vi "Batch_main_with_graph.vi"(1 "Stop":bool, 2 "ExpFilePath":path=path "D:/BaptisteData/BM13/CD1/data1/stabRF_exp_38.h5") -> ()   [LabVIEW 2013]
uses:
  <vilib>/addons/h5labview2/base/hid_t.ctl
  fpga-bitfile-ref.ctl
  host-subvis/Fast_sequence/sequence slot/slot-use.ctl
  host-subvis/Fast_sequence/sequence slot/triggers.ctl
  host-subvis/Fast_sequence/sequence slot/DAC.ctl
  host-subvis/Fast_sequence/sequence slot/DAC_fastseq-offset.ctl
  host-subvis/Fast_sequence/sequence slot/timing.ctl
  host-subvis/Fast_sequence/sequence slot/jump.ctl
  <vilib>/addons/h5labview2/file/H5Fmode.ctl
  <vilib>/addons/h5labview2/base/lib_path.vi
  <vilib>/addons/h5labview2/base/H5Equery.vi
  <vilib>/FPGAPlugInAG/sbRIO-9612/niLvFpga_Close_sbRIO-9612.vi
  <vilib>/addons/h5labview2/dataset/H5Dread.llb/H5Dread.xnode
  <vilib>/addons/h5labview2/attrib/H5Aread.llb/H5Aread.xnode
  <vilib>/rvi/interface/nirviCloseFPGA/nirviCloseFPGA.xnode
  FPGA Bitfiles/fpgabatch18_sbRIO9612RIO0_FPGAMAINMerlin_-1tLGtxjYvQ.lvbitx
  <vilib>/addons/h5labview2/attrib/H5Awrite.llb/H5Awrite.xnode
  <vilib>/addons/h5labview2/file/H5F.lvlib
  <vilib>/addons/h5labview2/dataset/H5D.lvlib
  <vilib>/addons/h5labview2/space/H5S.lvlib
panel:
  out "Remaning time (min)":dbl
  in  "temp file interval (ms)":i32=600
  in  "get variable interval (ms)":i32=300
  out "Graph":T1(graph)
  in  "Plot parameters":T2
  out "Temp data":sgl[][](array[numeric])
  out "Initial positions":T3(array[cluster])=[{"Name"="AWG", "kind"=7, "Value"=0.0}, {"Name"="Freq", "kind"=6, "Value"=2759965000.0}, {"Name"="Power", "kind"=6, "Value"=-40.0}, {"Name"="sus", "kind"=4, "Value"=0.29998779296875}, {"Name"="rus", "kind"=4, "Value"=0.29998779296875}, {"Name"="rls", "kind"=4, "Value"=0.29998779296875}, {"Name"="sls", "kind"=4, "Value"=0.059967041015625}, {"Name"="suq", "kind"=4, "Value"=-1.75994873046875}, {"Name"="suu", "kind"=4, "Value"=-0.749969482421875}, {"Name"="sur", "kind"=4, "Value"=-1.199951171875}, {"Name"="suc", "kind"=4, "Value"=-0.449981689453125}, {"Name"="sul", "kind"=4, "Value"=-0.89996337890625}, {"Name"="ruq", "kind"=4, "Value"=-1.699981689453125}, {"Name"="ruu", "kind"=4, "Value"=-0.749969482421875}, {"Name"="rur", "kind"=4, "Value"=-1.25}, {"Name"="ruc", "kind"=4, "Value"=-0.399932861328125}, {"Name"="rul", "kind"=4, "Value"=-0.89996337890625}, {"Name"="rlq", "kind"=4, "Value"=-1.7999267578125}, {"Name"="rlu", "kind"=4, "Value"=-0.89996337890625}, {"Name"="rlr", "kind"=4, "Value"=-1.199951171875}, {"Name"="rlc", "kind"=4, "Value"=-0.5999755859375}, {"Name"="rll", "kind"=4, "Value"=-0.749969482421875}, {"Name"="slq", "kind"=4, "Value"=-1.62506103515625}, {"Name"="slu", "kind"=4, "Value"=-0.89996337890625}, {"Name"="slr", "kind"=4, "Value"=-1.150054931640625}, {"Name"="slc", "kind"=4, "Value"=-0.449981689453125}, {"Name"="sll", "kind"=4, "Value"=-0.749969482421875}, {"Name"="tu", "kind"=4, "Value"=-0.89996337890625}, {"Name"="t", "kind"=4, "Value"=-0.89996337890625}, {"Name"="tl", "kind"=4, "Value"=-0.89996337890625}, {"Name"="4:7", "kind"=4, "Value"=-1.00006103515625}]
  in  "Buf size":i32=300
  out "Var index":u64[](array[numeric])=[0, 49, 0]
  out "start read vals":bool=TRUE
  out "Indexes File":u64[](array[numeric])=[8, 21, 0]
  out "Finish":bool=TRUE
  out "error out":errorcluster
  in  "File update interval (sec)":i32=3000000
  out "DAC_lock-in_info":T4={"Kind"=5, "Strings"=["DAC_Lock-in", "10.0.0.2", "V"], "uint64s"=[0, 1, 0, 0], "Doubles"=[1.0, 0.0, -1.0, -1.0, 50.0, 0.10000000149011612], "DAQmx take out list"=[]}
  out "Fast sequence parameters":T11={"Sequence size"=22, "IP address"="10.0.0.2", "Fast-seq-divider"=6661, "Trigger length"=300, "Sample count"=100, "Send all points?"=FALSE, "Upper limit"=1.0, "Lower limit"=-1.0, "Start ramp at"=0, "fast channels"=[{"dummy?"=FALSE, "panel"=0, "channel"=7}, {"dummy?"=FALSE, "panel"=1, "channel"=0}, {"dummy?"=FALSE, "panel"=0, "channel"=5}, {"dummy?"=FALSE, "panel"=1, "channel"=5}, {"dummy?"=FALSE, "panel"=1, "channel"=6}, {"dummy?"=FALSE, "panel"=1, "channel"=2}, {"dummy?"=FALSE, "panel"=2, "channel"=2}, {"dummy?"=FALSE, "panel"=2, "channel"=3}, {"dummy?"=FALSE, "panel"=2, "channel"=0}, {"dummy?"=FALSE, "panel"=2, "channel"=7}, {"dummy?"=FALSE, "panel"=3, "channel"=0}, {"dummy?"=FALSE, "panel"=2, "channel"=5}, {"dummy?"=FALSE, "panel"=3, "channel"=2}, {"dummy?"=FALSE, "panel"=3, "channel"=3}, {"dummy?"=FALSE, "panel"=3, "channel"=4}, {"dummy?"=FALSE, "panel"=4, "channel"=7}], "fastseq"=[{"use"=enum."triggers", "Triggers"={"triggers"={"1"=TRUE, "2"=TRUE, "3"=FALSE, "4"=FALSE}, "stop"=FALSE}, "DAC"={"FastChanNum"=0, "DAC offset"=0.0}, "timing"=0.0, "slot#"=0}, {"use"=enum."timing", "Triggers"={"triggers"={"1"=FALSE, "2"=FALSE, "3"=FALSE, "4"=FALSE}, "stop"=FALSE}, "DAC"={"FastChanNum"=0, "DAC offset"=0.0}, "timing"=1.0, "slot#"=0}, {"use"=enum."triggers", "Triggers"={"triggers"={"1"=TRUE, "2"=FALSE, "3"=FALSE, "4"=FALSE}, "stop"=FALSE}, "DAC"={"FastChanNum"=0, "DAC offset"=0.0}, "timing"=0.0, "slot#"=0}, {"use"=enum."timing", "Triggers"={"triggers"={"1"=FALSE, "2"=FALSE, "3"=FALSE, "4"=FALSE}, "stop"=FALSE}, "DAC"={"FastChanNum"=0, "DAC offset"=0.0}, "timing"=1.0, "slot#"=0}, {"use"=enum."DAC", "Triggers"={"triggers"={"1"=FALSE, "2"=FALSE, "3"=FALSE, "4"=FALSE}, "stop"=FALSE}, "DAC"={"FastChanNum"=1, "DAC offset"=0.0}, "timing"=0.0, "slot#"=0}, {"use"=enum."DAC", "Triggers"={"triggers"={"1"=FALSE, "2"=FALSE, "3"=FALSE, "4"=FALSE}, "stop"=FALSE}, "DAC"={"FastChanNum"=0, "DAC offset"=0.0}, "timing"=0.0, "slot#"=0}, {"use"=enum."DAC", "Triggers"={"triggers"={"1"=FALSE, "2"=FALSE, "3"=FALSE, "4"=FALSE}, "stop"=FALSE}, "DAC"={"FastChanNum"=4, "DAC offset"=0.0}, "timing"=0.0, "slot#"=0}, {"use"=enum."DAC", "Triggers"={"triggers"={"1"=FALSE, "2"=FALSE, "3"=FALSE, "4"=FALSE}, "stop"=FALSE}, "DAC"={"FastChanNum"=3, "DAC offset"=0.0}, "timing"=0.0, "slot#"=0}, {"use"=enum."DAC", "Triggers"={"triggers"={"1"=FALSE, "2"=FALSE, "3"=FALSE, "4"=FALSE}, "stop"=FALSE}, "DAC"={"FastChanNum"=7, "DAC offset"=0.0}, "timing"=0.0, "slot#"=0}, {"use"=enum."DAC", "Triggers"={"triggers"={"1"=FALSE, "2"=FALSE, "3"=FALSE, "4"=FALSE}, "stop"=FALSE}, "DAC"={"FastChanNum"=6, "DAC offset"=0.0}, "timing"=0.0, "slot#"=0}, {"use"=enum."DAC", "Triggers"={"triggers"={"1"=FALSE, "2"=FALSE, "3"=FALSE, "4"=FALSE}, "stop"=FALSE}, "DAC"={"FastChanNum"=10, "DAC offset"=0.0}, "timing"=0.0, "slot#"=0}, {"use"=enum."DAC", "Triggers"={"triggers"={"1"=FALSE, "2"=FALSE, "3"=FALSE, "4"=FALSE}, "stop"=FALSE}, "DAC"={"FastChanNum"=9, "DAC offset"=0.0}, "timing"=0.0, "slot#"=0}, {"use"=enum."timing", "Triggers"={"triggers"={"1"=FALSE, "2"=FALSE, "3"=FALSE, "4"=FALSE}, "stop"=FALSE}, "DAC"={"FastChanNum"=0, "DAC offset"=0.0}, "timing"=10.0, "slot#"=0}, {"use"=enum."DAC", "Triggers"={"triggers"={"1"=FALSE, "2"=FALSE, "3"=FALSE, "4"=FALSE}, "stop"=FALSE}, "DAC"={"FastChanNum"=1, "DAC offset"=0.0}, "timing"=0.0, "slot#"=0}, {"use"=enum."DAC", "Triggers"={"triggers"={"1"=FALSE, "2"=FALSE, "3"=FALSE, "4"=FALSE}, "stop"=FALSE}, "DAC"={"FastChanNum"=0, "DAC offset"=0.0}, "timing"=0.0, "slot#"=0}, {"use"=enum."DAC", "Triggers"={"triggers"={"1"=FALSE, "2"=FALSE, "3"=FALSE, "4"=FALSE}, "stop"=FALSE}, "DAC"={"FastChanNum"=4, "DAC offset"=0.0}, "timing"=0.0, "slot#"=0}, {"use"=enum."DAC", "Triggers"={"triggers"={"1"=FALSE, "2"=FALSE, "3"=FALSE, "4"=FALSE}, "stop"=FALSE}, "DAC"={"FastChanNum"=3, "DAC offset"=0.0}, "timing"=0.0, "slot#"=0}, {"use"=enum."DAC", "Triggers"={"triggers"={"1"=FALSE, "2"=FALSE, "3"=FALSE, "4"=FALSE}, "stop"=FALSE}, "DAC"={"FastChanNum"=7, "DAC offset"=0.0}, "timing"=0.0, "slot#"=0}, {"use"=enum."DAC", "Triggers"={"triggers"={"1"=FALSE, "2"=FALSE, "3"=FALSE, "4"=FALSE}, "stop"=FALSE}, "DAC"={"FastChanNum"=6, "DAC offset"=0.0}, "timing"=0.0, "slot#"=0}, {"use"=enum."DAC", "Triggers"={"triggers"={"1"=FALSE, "2"=FALSE, "3"=FALSE, "4"=FALSE}, "stop"=FALSE}, "DAC"={"FastChanNum"=10, "DAC offset"=0.0}, "timing"=0.0, "slot#"=0}, {"use"=enum."DAC", "Triggers"={"triggers"={"1"=FALSE, "2"=FALSE, "3"=FALSE, "4"=FALSE}, "stop"=FALSE}, "DAC"={"FastChanNum"=9, "DAC offset"=0.0}, "timing"=0.0, "slot#"=0}, {"use"=enum."jump", "Triggers"={"triggers"={"1"=FALSE, "2"=FALSE, "3"=FALSE, "4"=FALSE}, "stop"=FALSE}, "DAC"={"FastChanNum"=0, "DAC offset"=0.0}, "timing"=0.0, "slot#"=21}]} {"fastseq"."DAC"."DAC offset" min=-1 max=0.5; "fastseq"."DAC"."FastChanNum" max=15 step=1; "fastseq"."slot#" max=4095}
  out "Timings":dbl[][](array[numeric])=[[2417234066.0, 52858.0]] format="%^#_4g"
  out "Indexes":i32[](array[numeric])=[8, 21, 0]
  out "sweep_dim":u64[](array[numeric])=[11, 61, 61]
  out "Readout parameters":T12(array[cluster])=[{"Kind"=0, "Strings"=["ADC", "", "V", "sud;rud;rld;sld", "nA;nA;nA;nA", "100.0;100.0;100.0;100.0"], "uint64s"=[5, 4, 250000, 1, 100, 10106, 1000000, 10000, 0, 1], "Doubles"=[1.0], "DAQmx take out list"=["", ""]}]
  out "Exp_params":T15={"filename"="201612181913", "ExpFilePath"=path "C:/Documents and Settings/Bauerle/Mes documents/takada/HBT6/201612181913.h5", "File Ref list"=[16777217, 33554433, 16777216, 33554432], "sweep_dim"=[11, 61, 61], "sweep_list"=["suq", "ruq", "rlq", "slq", "sur", "rur", "rlr", "slr", "suc", "ruc", "rlc", "slc"], "readout_list"=["sud", "rud", "rld", "sld"], "Sweep instrument bools"=[[0, 0], [0, 0], [0, 0], [0, 0], [0, 0], [0, 0], [0, 0], [0, 0], [0, 0], [0, 0], [0, 0], [0, 0], [0, 0], [0, 0], [0, 0], [0, 0], [0, 0], [0, 0], [0, 0], [0, 0], [0, 0], [0, 0], [0, 0], [0, 0], [0, 0], [0, 0], [0, 0], [0, 0], [0, 0], [0, 0], [0, 0], [0, 0], [0, 0], [0, 0], [0, 0], [0, 0], [0, 0], [0, 0], [0, 0], [0, 0], [0, 0]], "Read out instrument bools"=[[1, 0]], "Experimental bool list"=[TRUE, TRUE], "Initial move"=[{"Name"="None", "kind"=100, "Value"=0.0}], "FPGA Ref"=refnum, "Inst_parameters"={"ConfigFilePath"=path "\\\\10.0.0.7\\takada2/DATA/HBT6/data/Configs/conf_20161218_fc_load.h5", "Inst_list"=["ADC", "AWG", "Freq", "Power", "sus", "rus", "rls", "sls", "suq", "suu", "sur", "suc", "sul", "ruq", "ruu", "rur", "ruc", "rul", "rlq", "rlu", "rlr", "rlc", "rll", "slq", "slu", "slr", "slc", "sll", "tu", "t", "tl", "fast_sequence", "4:7", "suc_load", "sur_load", "ruc_load", "rur_load", "rlc_load", "rlr_load", "slc_load", "slr_load", "load_time"], "fast_mode"=[1, 0], "Wait_times"=[1, 1, 1, 1], "Inst_array"=[{"Kind"=0, "Strings"=["ADC", "", "V", "sud;rud;rld;sld", "nA;nA;nA;nA", "100.0;100.0;100.0;100.0"], "uint64s"=[5, 4, 250000, 1, 100, 10106, 1000000, 1, 0, 1], "Doubles"=[1.0], "DAQmx take out list"=[]}, {"Kind"=7, "Strings"=["AWG", "10.0.0.4", "", "C:\\Documents and Settings\\Bauerle\\Mes documents\\Bautze\\FPGA-clean_works_1.13.6_batchtest\\Python\\AWG", "dummy", "SAWnstrig_v4.py"], "uint64s"=[2, 0, 0, 3, 0, 0, 0, 0, 0, 0, 0, 0, 0, 0], "Doubles"=[1200000000.0, 1.0, 0.0, 1.0, 0.0, 1.0, 0.0, 1.0, 0.0, 1.0, 0.0, 1.0, 0.0], "DAQmx take out list"=[]}, {"Kind"=6, "Strings"=["Freq", "0:19", "GHz"], "uint64s"=[1, 0, 0, 0, 2, 0, 0, 0], "Doubles"=[2.0, -30.0, 200.0, 100.0, 0.0, 6.000999927520752, 9.000000318337698e-06, 30.0, -145.0], "DAQmx take out list"=[]}, {"Kind"=6, "Strings"=["Power", "0:19", "GHz"], "uint64s"=[1, 0, 1, 0, 2, 0, 0, 1], "Doubles"=[2.0, -30.0, 200.0, 100.0, 0.0, 6.000999927520752, 9.000000318337698e-06, 30.0, -145.0], "DAQmx take out list"=[]}, {"Kind"=4, "Strings"=["sus", "10.0.0.2", "mV"], "uint64s"=[0, 1], "Doubles"=[1.0, -1.0, 1.0, -1.0, 1.0], "DAQmx take out list"=[]}, {"Kind"=4, "Strings"=["rus", "10.0.0.2", "mV"], "uint64s"=[0, 2], "Doubles"=[1.0, -1.0, 1.0, -1.0, 1.0], "DAQmx take out list"=[]}, {"Kind"=4, "Strings"=["rls", "10.0.0.2", "mV"], "uint64s"=[0, 3], "Doubles"=[1.0, -1.0, 1.0, -1.0, 1.0], "DAQmx take out list"=[]}, {"Kind"=4, "Strings"=["sls", "10.0.0.2", "mV"], "uint64s"=[0, 4], "Doubles"=[1.0, -1.0, 1.0, -1.0, 1.0], "DAQmx take out list"=[]}, {"Kind"=4, "Strings"=["suq", "10.0.0.2", "V"], "uint64s"=[0, 5], "Doubles"=[0.30000001192092896, -2.0, 1.0, -1.0, 1.0], "DAQmx take out list"=[]}, {"Kind"=4, "Strings"=["suu", "10.0.0.2", "V"], "uint64s"=[0, 6], "Doubles"=[0.30000001192092896, -2.0, 1.0, -1.0, 1.0], "DAQmx take out list"=[]}, {"Kind"=4, "Strings"=["sur", "10.0.0.2", "V"], "uint64s"=[0, 7], "Doubles"=[0.30000001192092896, -2.0, 1.0, -1.0, 1.0], "DAQmx take out list"=[]}, {"Kind"=4, "Strings"=["suc", "10.0.0.2", "V"], "uint64s"=[1, 0], "Doubles"=[0.30000001192092896, -2.0, 1.0, -1.0, 1.0], "DAQmx take out list"=[]}, {"Kind"=4, "Strings"=["sul", "10.0.0.2", "V"], "uint64s"=[1, 1], "Doubles"=[0.30000001192092896, -2.0, 1.0, -1.0, 1.0], "DAQmx take out list"=[]}, {"Kind"=4, "Strings"=["ruq", "10.0.0.2", "V"], "uint64s"=[1, 2], "Doubles"=[0.30000001192092896, -2.0, 1.0, -1.0, 1.0], "DAQmx take out list"=[]}, {"Kind"=4, "Strings"=["ruu", "10.0.0.2", "V"], "uint64s"=[1, 3], "Doubles"=[0.30000001192092896, -2.0, 1.0, -1.0, 1.0], "DAQmx take out list"=[]}, {"Kind"=4, "Strings"=["rur", "10.0.0.2", "V"], "uint64s"=[1, 5], "Doubles"=[0.30000001192092896, -2.0, 1.0, -1.0, 1.0], "DAQmx take out list"=[]}, {"Kind"=4, "Strings"=["ruc", "10.0.0.2", "V"], "uint64s"=[1, 6], "Doubles"=[0.30000001192092896, -2.0, 1.0, -1.0, 1.0], "DAQmx take out list"=[]}, {"Kind"=4, "Strings"=["rul", "10.0.0.2", "V"], "uint64s"=[1, 7], "Doubles"=[0.30000001192092896, -2.0, 1.0, -1.0, 1.0], "DAQmx take out list"=[]}, {"Kind"=4, "Strings"=["rlq", "10.0.0.2", "V"], "uint64s"=[2, 0], "Doubles"=[0.30000001192092896, -2.0, 1.0, -1.0, 1.0], "DAQmx take out list"=[]}, {"Kind"=4, "Strings"=["rlu", "10.0.0.2", "V"], "uint64s"=[2, 1], "Doubles"=[0.30000001192092896, -2.0, 1.0, -1.0, 1.0], "DAQmx take out list"=[]}, {"Kind"=4, "Strings"=["rlr", "10.0.0.2", "V"], "uint64s"=[2, 2], "Doubles"=[0.30000001192092896, -2.0, 1.0, -1.0, 1.0], "DAQmx take out list"=[]}, {"Kind"=4, "Strings"=["rlc", "10.0.0.2", "V"], "uint64s"=[2, 3], "Doubles"=[0.30000001192092896, -2.0, 1.0, -1.0, 1.0], "DAQmx take out list"=[]}, {"Kind"=4, "Strings"=["rll", "10.0.0.2", "V"], "uint64s"=[2, 4], "Doubles"=[0.30000001192092896, -2.0, 1.0, -1.0, 1.0], "DAQmx take out list"=[]}, {"Kind"=4, "Strings"=["slq", "10.0.0.2", "V"], "uint64s"=[2, 5], "Doubles"=[0.30000001192092896, -2.0, 1.0, -1.0, 1.0], "DAQmx take out list"=[]}, {"Kind"=4, "Strings"=["slu", "10.0.0.2", "V"], "uint64s"=[2, 6], "Doubles"=[0.30000001192092896, -2.0, 1.0, -1.0, 1.0], "DAQmx take out list"=[]}, {"Kind"=4, "Strings"=["slr", "10.0.0.2", "V"], "uint64s"=[2, 7], "Doubles"=[0.30000001192092896, -2.0, 1.0, -1.0, 1.0], "DAQmx take out list"=[]}, {"Kind"=4, "Strings"=["slc", "10.0.0.2", "V"], "uint64s"=[3, 0], "Doubles"=[0.30000001192092896, -2.0, 1.0, -1.0, 1.0], "DAQmx take out list"=[]}, {"Kind"=4, "Strings"=["sll", "10.0.0.2", "V"], "uint64s"=[3, 1], "Doubles"=[0.30000001192092896, -2.0, 1.0, -1.0, 1.0], "DAQmx take out list"=[]}, {"Kind"=4, "Strings"=["tu", "10.0.0.2", "V"], "uint64s"=[3, 2], "Doubles"=[0.30000001192092896, -2.0, 1.0, -1.0, 1.0], "DAQmx take out list"=[]}, {"Kind"=4, "Strings"=["t", "10.0.0.2", "V"], "uint64s"=[3, 3], "Doubles"=[0.30000001192092896, -2.0, 1.0, -1.0, 1.0], "DAQmx take out list"=[]}, {"Kind"=4, "Strings"=["tl", "10.0.0.2", "V"], "uint64s"=[3, 4], "Doubles"=[0.30000001192092896, -2.0, 1.0, -1.0, 1.0], "DAQmx take out list"=[]}, {"Kind"=9, "Strings"=["fast_sequence", "10.0.0.2", "V"], "uint64s"=[6661, 300, 100, 0, 7, 8, 5, 13, 14, 10, 18, 19, 16, 23, 24, 21, 26, 27, 28, 39, 0], "Doubles"=[1.0, -1.0, -1.0, -1.0], "DAQmx take out list"=[]}, {"Kind"=4, "Strings"=["4:7", "10.0.0.2", "V"], "uint64s"=[4, 7], "Doubles"=[0.30000001192092896, -2.0, 1.0, -1.0, 1.0], "DAQmx take out list"=[]}, {"Kind"=10, "Strings"=["suc_load", "10.0.0.2", "V"], "uint64s"=[4, 0], "Doubles"=[0.5, -0.5], "DAQmx take out list"=[]}, {"Kind"=10, "Strings"=["sur_load", "10.0.0.2", "V"], "uint64s"=[5, 0], "Doubles"=[0.5, -0.5], "DAQmx take out list"=[]}, {"Kind"=10, "Strings"=["ruc_load", "10.0.0.2", "V"], "uint64s"=[6, 0], "Doubles"=[0.5, -0.5], "DAQmx take out list"=[]}, {"Kind"=10, "Strings"=["rur_load", "10.0.0.2", "V"], "uint64s"=[7, 0], "Doubles"=[0.5, -0.5], "DAQmx take out list"=[]}, {"Kind"=10, "Strings"=["rlc_load", "10.0.0.2", "V"], "uint64s"=[8, 0], "Doubles"=[0.5, -0.5], "DAQmx take out list"=[]}, {"Kind"=10, "Strings"=["rlr_load", "10.0.0.2", "V"], "uint64s"=[9, 0], "Doubles"=[0.5, -0.5], "DAQmx take out list"=[]}, {"Kind"=10, "Strings"=["slc_load", "10.0.0.2", "V"], "uint64s"=[10, 0], "Doubles"=[0.5, -0.5], "DAQmx take out list"=[]}, {"Kind"=10, "Strings"=["slr_load", "10.0.0.2", "V"], "uint64s"=[11, 0], "Doubles"=[0.5, -0.5], "DAQmx take out list"=[]}, {"Kind"=10, "Strings"=["load_time", "10.0.0.2", "ms"], "uint64s"=[12, 0], "Doubles"=[1000.0, -0.009999999776482582], "DAQmx take out list"=[]}]}} {"File Ref list" format="%.0x"}
  out "Sweep inst info":T12(array[cluster])=[{"Kind"=4, "Strings"=["suq", "10.0.0.2", "V"], "uint64s"=[0, 5], "Doubles"=[0.30000001192092896, -2.0, 1.0, -1.0, 1.0], "DAQmx take out list"=[]}, {"Kind"=4, "Strings"=["ruq", "10.0.0.2", "V"], "uint64s"=[1, 2], "Doubles"=[0.30000001192092896, -2.0, 1.0, -1.0, 1.0], "DAQmx take out list"=[]}, {"Kind"=4, "Strings"=["rlq", "10.0.0.2", "V"], "uint64s"=[2, 0], "Doubles"=[0.30000001192092896, -2.0, 1.0, -1.0, 1.0], "DAQmx take out list"=[]}, {"Kind"=4, "Strings"=["slq", "10.0.0.2", "V"], "uint64s"=[2, 5], "Doubles"=[0.30000001192092896, -2.0, 1.0, -1.0, 1.0], "DAQmx take out list"=[]}, {"Kind"=4, "Strings"=["sur", "10.0.0.2", "V"], "uint64s"=[0, 7], "Doubles"=[0.30000001192092896, -2.0, 1.0, -1.0, 1.0], "DAQmx take out list"=[]}, {"Kind"=4, "Strings"=["rur", "10.0.0.2", "V"], "uint64s"=[1, 5], "Doubles"=[0.30000001192092896, -2.0, 1.0, -1.0, 1.0], "DAQmx take out list"=[]}, {"Kind"=4, "Strings"=["rlr", "10.0.0.2", "V"], "uint64s"=[2, 2], "Doubles"=[0.30000001192092896, -2.0, 1.0, -1.0, 1.0], "DAQmx take out list"=[]}, {"Kind"=4, "Strings"=["slr", "10.0.0.2", "V"], "uint64s"=[2, 7], "Doubles"=[0.30000001192092896, -2.0, 1.0, -1.0, 1.0], "DAQmx take out list"=[]}, {"Kind"=4, "Strings"=["suc", "10.0.0.2", "V"], "uint64s"=[1, 0], "Doubles"=[0.30000001192092896, -2.0, 1.0, -1.0, 1.0], "DAQmx take out list"=[]}, {"Kind"=4, "Strings"=["ruc", "10.0.0.2", "V"], "uint64s"=[1, 6], "Doubles"=[0.30000001192092896, -2.0, 1.0, -1.0, 1.0], "DAQmx take out list"=[]}, {"Kind"=4, "Strings"=["rlc", "10.0.0.2", "V"], "uint64s"=[2, 3], "Doubles"=[0.30000001192092896, -2.0, 1.0, -1.0, 1.0], "DAQmx take out list"=[]}, {"Kind"=4, "Strings"=["slc", "10.0.0.2", "V"], "uint64s"=[3, 0], "Doubles"=[0.30000001192092896, -2.0, 1.0, -1.0, 1.0], "DAQmx take out list"=[]}]
  # "total"
  # "nb of calls"
  # "average"
  # "total time"
  # "read config"
  # "plot loop"
  # "save data"
  # "config instr"
  # "FPGA init"
  # "voltmeter init"
  # "initial move"
  # "read init values"
  # "meas loop"
  # "move + wait"
  # "FPGA config"
  # "FPGA start"
  # "FPGA stop"
  # "read data"
  # "clear buffer"
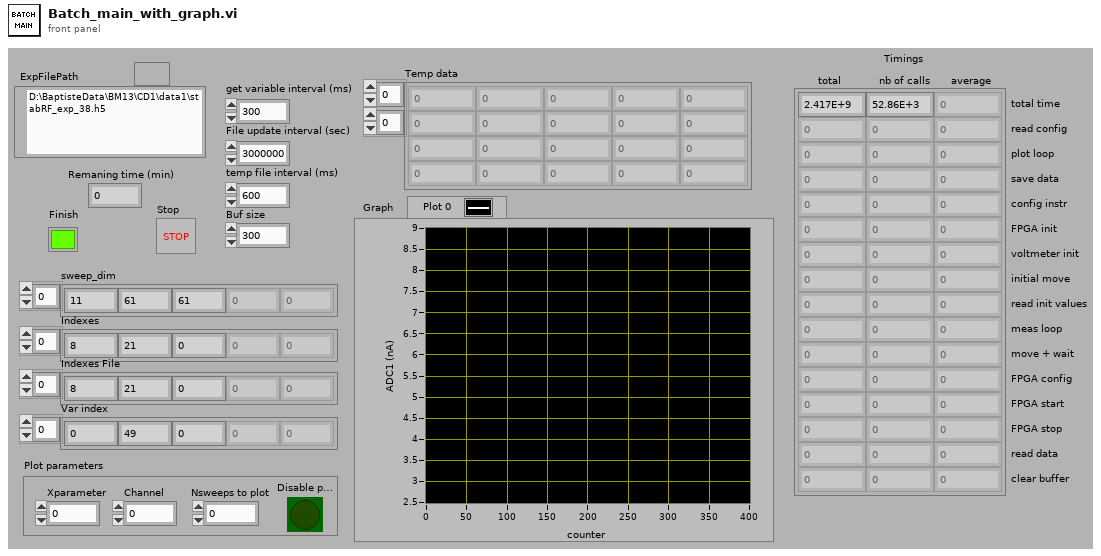
[diagram p1: front panel]
types:
  T1 = cluster{"Sweep buffer":dbl[], "Readout buffer":dbl[]}
  T2 = cluster{"Disable plot":bool, "Nsweeps to plot":dbl, "Channel":dbl, "Xparameter":dbl, "Readout buffer":dbl[][], "Sweep buffer":dbl[][]}
  T3 = cluster{"Name":string, "kind":u64, "Value":dbl}[]
  T4 = cluster{"Kind":u16, "Strings":string[], "uint64s":u64[], "Doubles":dbl[], "DAQmx take out list":refnum<k21>[]}
  T5 = typedef "slot-use.ctl" = enum8{"DAC", "timing", "triggers", "jump"}
  T6 = typedef "triggers.ctl" = cluster{"triggers":cluster{"1":bool, "2":bool, "3":bool, "4":bool}, "stop":bool}
  T7 = typedef "DAC.ctl" = cluster{"FastChanNum":u8, "DAC offset":T8}
  T8 = typedef "DAC_fastseq-offset.ctl" = sgl
  T9 = typedef "timing.ctl" = sgl
  T10 = typedef "jump.ctl" = u16
  T11 = cluster{"Sequence size":u64, "IP address":string, "Fast-seq-divider":u64, "Trigger length":u64, "Sample count":u64, "Send all points?":bool, "Upper limit":dbl, "Lower limit":dbl, "Start ramp at":u64, "fast channels":cluster{"dummy?":bool, "panel":u8, "channel":u8}[], "fastseq":cluster{"use":T5, "Triggers":T6, "DAC":T7, "timing":T9, "slot#":T10}[]}
  T12 = cluster{"Kind":u16, "Strings":string[], "uint64s":u64[], "Doubles":dbl[], "DAQmx take out list":refnum<k21>[]}[]
  T13 = typedef "hid_t.ctl" = i32
  T14 = typedef "fpga-bitfile-ref.ctl" = refnum<k20>
  T15 = cluster{"filename":string, "ExpFilePath":path, "File Ref list":T13[], "sweep_dim":u64[], "sweep_list":string[], "readout_list":string[], "Sweep instrument bools":u64[][], "Read out instrument bools":u64[][], "Experimental bool list":bool[], "Initial move":cluster{"Name":string, "kind":u64, "Value":dbl}[], "FPGA Ref":T14, "Inst_parameters":cluster{"ConfigFilePath":path, "Inst_list":string[], "fast_mode":u8[], "Wait_times":u64[], "Inst_array":cluster{"Kind":u16, "Strings":string[], "uint64s":u64[], "Doubles":dbl[], "DAQmx take out list":refnum<k21>[]}[]}}
  T16 = cluster{"filename":string, "ExpFilePath":path, "File Ref list":T13[], "sweep_dim":u64[], "sweep_list":string[], "readout_list":string[], "Sweep instrument bools":u64[][], "Read out instrument bools":u64[][], "Experimental bool list":bool[], "Initial moves":cluster{"name":string, "parameter":u64, "value":dbl}[], "FPGA Ref":T14, "Inst_parameters":cluster{"ConfigFilePath":path, "Inst_list":string[], "fast_mode":u8[], "Wait_times":u64[], "Inst_array":cluster{"Kind":u16, "Strings":string[], "uint64s":u64[], "Doubles":dbl[], "DAQmx take out list":refnum<k21>[]}[]}}
  T17 = typedef "H5F.lvlib/H5Fmode.ctl" = enum16{"read-only", "read-write", "overwrite", "create new", "open or create"}
  T18 = enum16{"stop", "set divider", "unset ramp mode", "unset stop count", "set pulse lenght", "set ramp", "start"}
  T19 = cluster{"Kind":u16, "Strings":string[], "uint64s":u64[], "Doubles":dbl[], refnum<k21>[]}[]
  T20 = cluster{"use":T5, "Triggers":T6, "DAC":T7, "timing":T9, "slot#":T10}[]
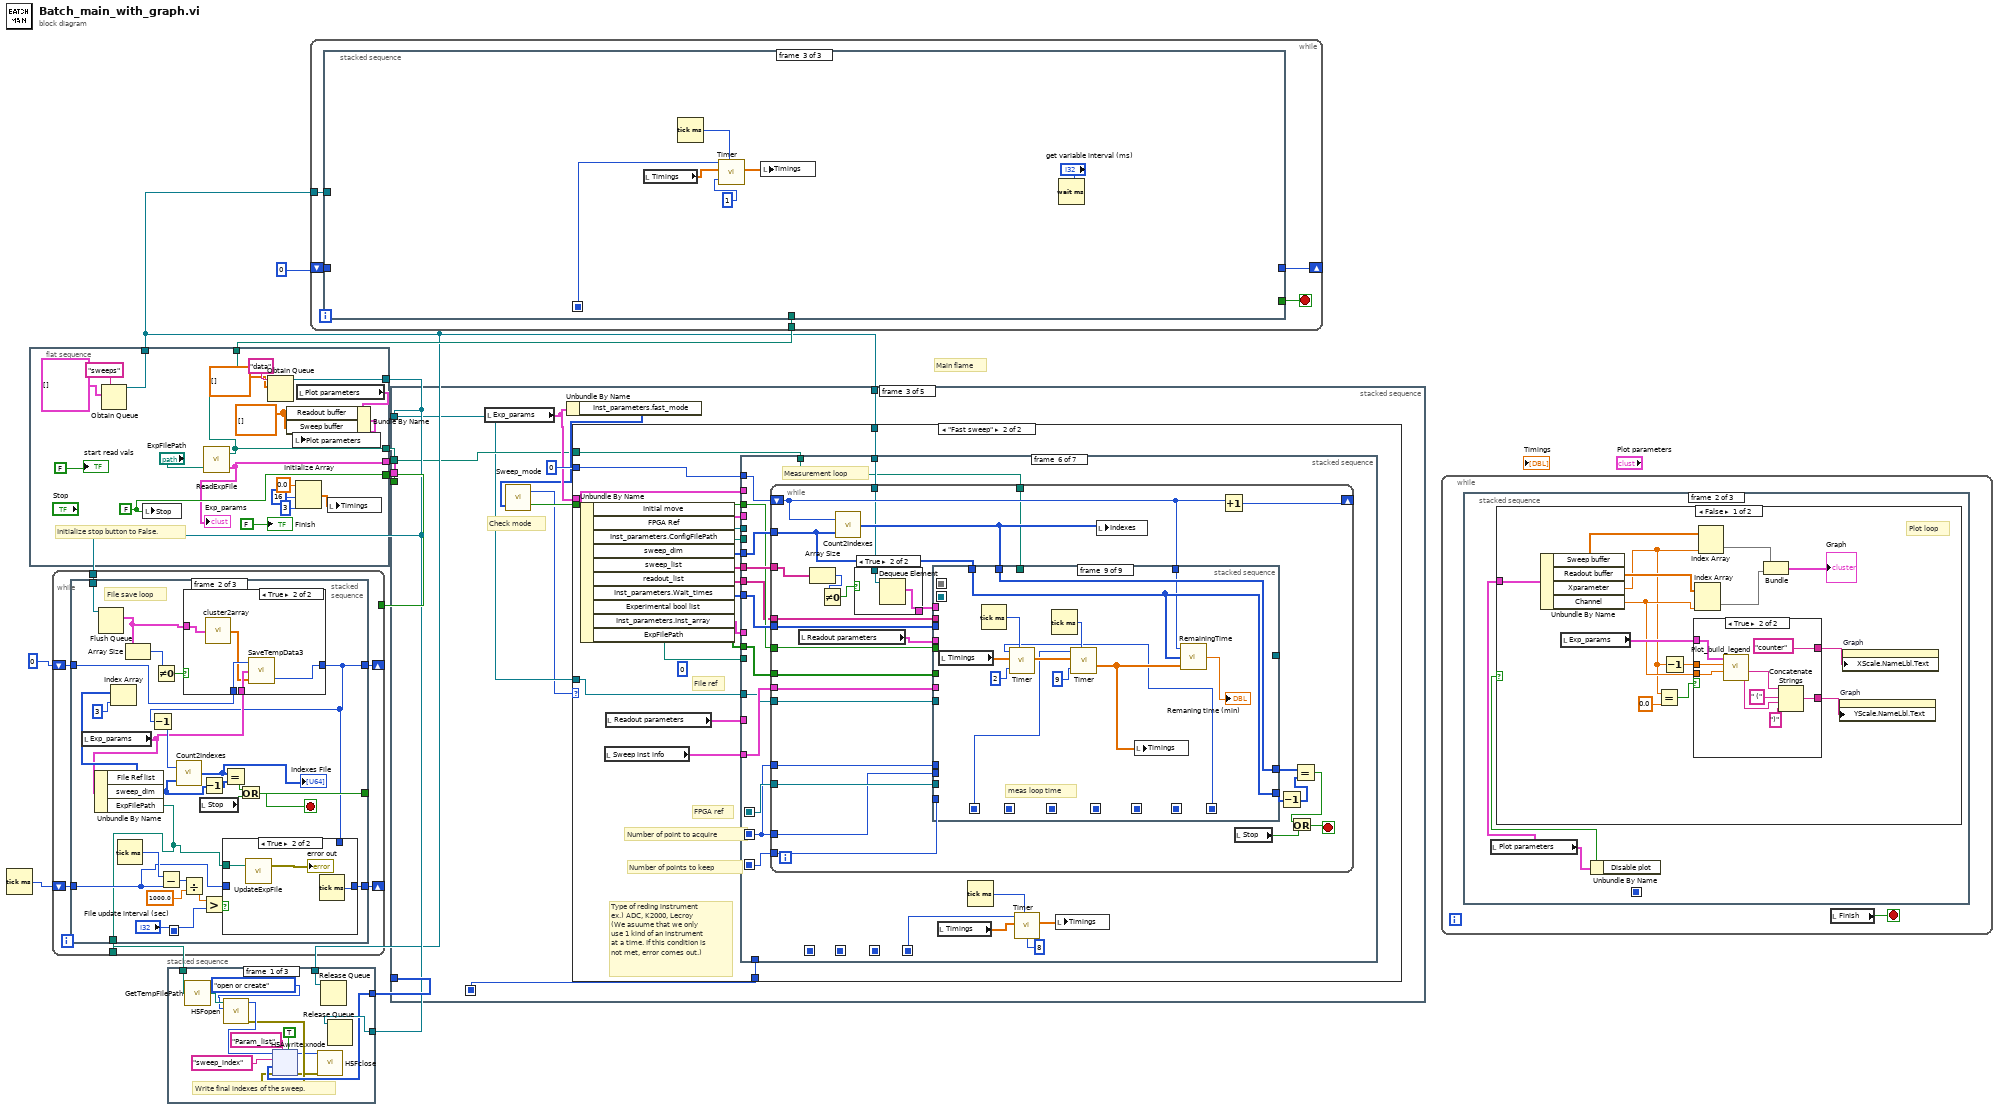
[diagram p0: block diagram]
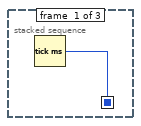
[diagram p2: hidden frame]
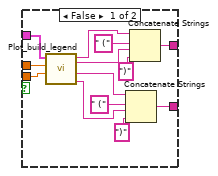
[diagram p3: hidden frame]
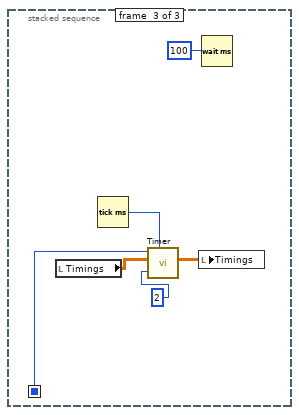
[diagram p5: hidden frame]
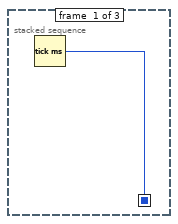
[diagram p6: hidden frame]
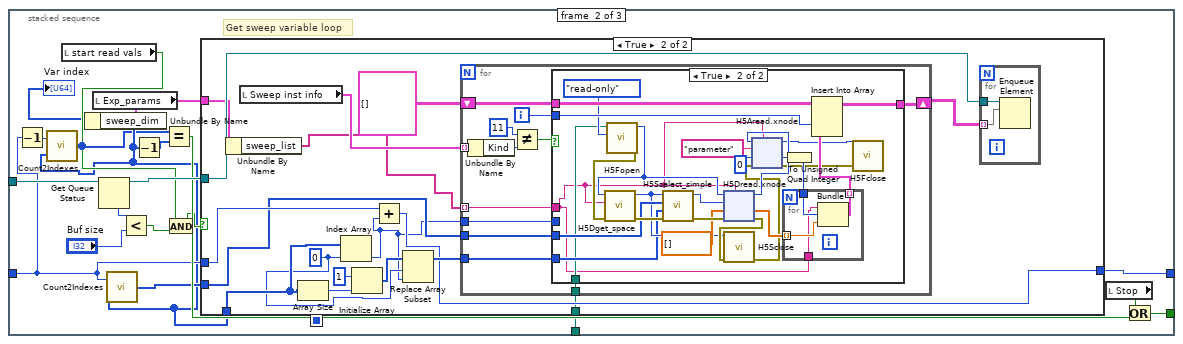
[diagram p7: hidden frame]
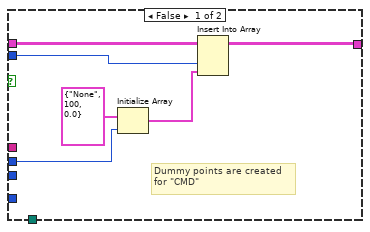
[diagram p9: hidden frame]
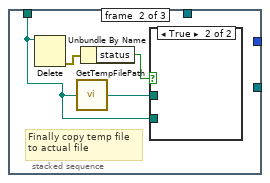
[diagram p10: hidden frame]
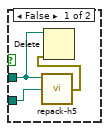
[diagram p11: hidden frame]
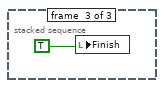
[diagram p12: hidden frame]
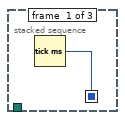
[diagram p13: hidden frame]
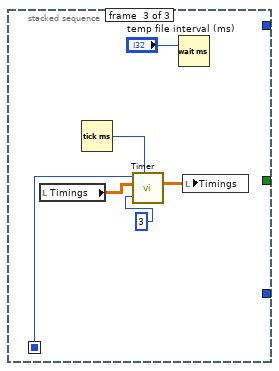
[diagram p16: hidden frame]
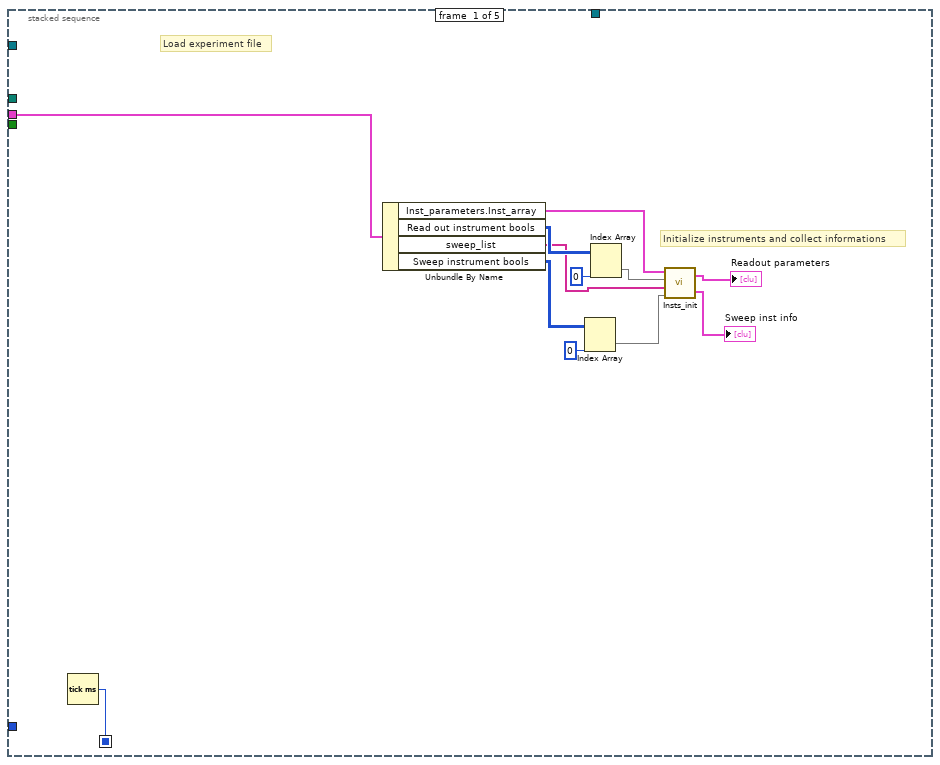
[diagram p17: hidden frame]
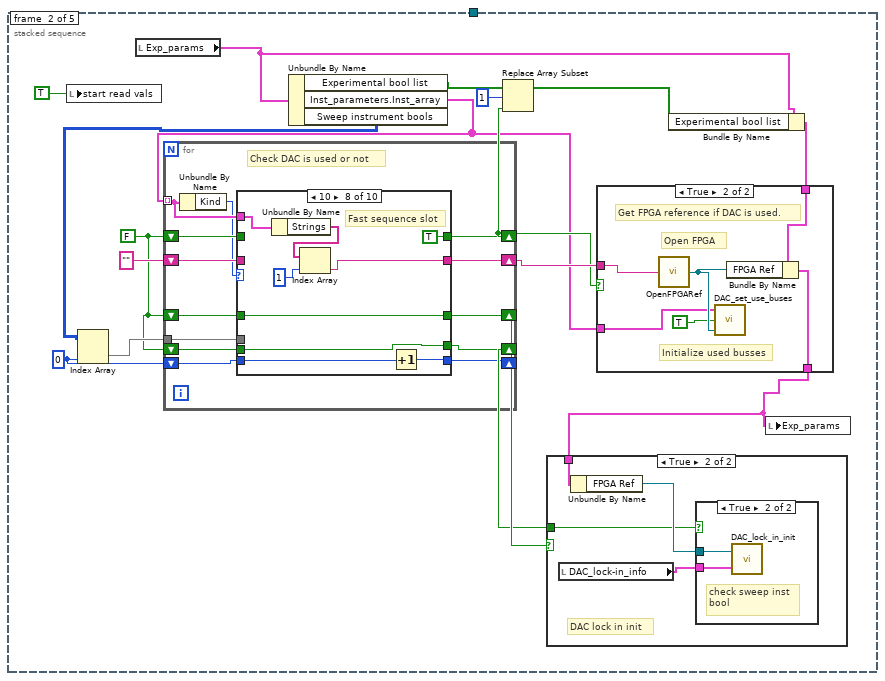
[diagram p18: hidden frame]
diagram:
  # "Main flame"
  n1 = Tick Count (ms)() -> (millisecond timer value=w10:u32)
  n2 = flat-sequence {
    tunnel: [w30] -> w7
    tunnel: [w21] -> w2
    tunnel: [w25] -> w1
    tunnel: [w22] -> w5
    tunnel: [w18] -> w4
    tunnel: [w18] -> w3
    frame #0 {
      w19 = dbl[][] []
      w30 = FALSE
      # "Initialize stop button to False."
      n3 = Obtain Queue(name (unnamed)="sweeps", element data type=cluster{string, "data":u64, dbl}[] []) -> (queue out=w25:refnum<queue>)  [unwired: 3 in, 2 out]
      n4 = local write "Stop"(w30) -> ()
      n5 = call "ReadExpFile.vi"("ExpFilePath"="ExpFilePath") -> ("Exp_params"=w22:T16, "WorkFilePath"=w18:path)  [unwired: 1 in]
      "Exp_params" <- w22
      n6 = Obtain Queue(name (unnamed)="data", element data type=dbl[][] []) -> (queue out=w21:refnum<queue>)  [unwired: 3 in, 2 out]
      n7 = Initialize Array(0.0, 16, 3) -> (w14:dbl[][])
      n8 = local read "Plot parameters"() -> (w16:T2)
      n9 = Bundle By Name(cluster=w16, "Readout buffer"=w19, "Sweep buffer"=w19) -> (w17:T2)
      n10 = local write "Plot parameters"(w17) -> ()
      n11 = local write "Timings"(w14) -> ()
      "Finish" <- FALSE
      "start read vals" <- FALSE
    }
  }
  n12 = while {
    shift-right: [w31] -> _
    shift-left: 0 -> [w36]
    shift-right: [w34] -> _
    shift-left: w10 -> [w35]
    tunnel: [w32] -> w8
    tunnel: w7 -> [_]
    tunnel: w2 -> [w33]
    stop <- w37 stop-if-true
    n13 = stacked-sequence {
      seq-local: [w38 _ _] -> [_ _ w78]
      tunnel: [_ w59 _] -> w37
      tunnel: w36 -> [_ w57 _]
      tunnel: w35 -> [_ w48 _]
      tunnel: [_ w47 _] -> w34
      tunnel: w33 -> [_ w41 _]
      tunnel: [_ w40 _] -> w32
      tunnel: [_ w39 _] -> w31
      frame #0 {
        n14 = Tick Count (ms)() -> (millisecond timer value=w38:u32)
      }
      frame #1 {
        # "File save loop"
        n15 = local read "Exp_params"() -> (w44:T15)
        n16 = Unbundle By Name(w44) -> ("File Ref list"=w45:T13[], "sweep_dim"=w60:u64[], "ExpFilePath"=w40:path)
        n17 = Flush Queue(queue=w41) -> (remaining elements=w42:cluster{dbl[][]}[])  [unwired: 1 in, 2 out]
        n18 = Index Array(array=w45, index=3) -> ()  [unwired: 1 out]
        n19 = Tick Count (ms)() -> (millisecond timer value=w55:u32)
        n20 = Array Size(array=w42) -> (size(s)=w43:i32)
        n21 = Not Equal To 0?(x=w43) -> (x != 0?=w58:bool)
        n22 = Subtract(x=w55, y=w48) -> (x-y=w54:u32)
        n23 = Divide(x=w54, y=1000.0) -> (x/y=w52:dbl)
        n24 = case shown="True" w58 {
          tunnel: w57 -> [w68 w73]
          tunnel: [w68 w72] -> w39
          tunnel: w44 -> [_ w71]
          tunnel: w42 -> [_ w70]
          frame False {
          }
          frame True {
            n25 = call "cluster2array.vi"("temp data"=w70) -> ("temp data array"=w69:dbl[][][])
            n26 = call "SaveTempData3.vi"("temp data"=w69, "Exp_params"=w71, "count"=w73) -> ("count out"=w72:i32)  [unwired: 1 in]
          }
        }
        n27 = Decrement(x=w39) -> (x-1=w56:i32)
        n28 = call "Count2Indexes.vi"("sweep_dim"=w60, "Count"=w56) -> ("Indexes"=w49:u64[])
        "Indexes File" <- w49
        n29 = local read "Stop"() -> (w63:bool)
        n30 = Decrement(x=w60) -> (x-1=w61:u64[])
        n31 = Greater?(x=w52, y="File update interval (sec)") -> (0:w50:bool)
        n32 = Equal?(x=w49, y=w61) -> (x = y?=w62:bool)
        n33 = case shown="True" w50 {
          tunnel: w48 -> [w64 _]
          tunnel: [w64 w66] -> w47
          tunnel: w40 -> [_ w65]
          tunnel: w39 -> [_ _]
          frame False {
          }
          frame True {
            n34 = call "UpdateExpFile.vi"("ExpFilePath"=w65) -> ("error out"=→"error out":errorcluster)  [unwired: 2 in]
            n35 = Tick Count (ms)() -> (millisecond timer value=w66:u32)
          }
        }
        n36 = Or(x=w62, y=w63) -> (x .or. y?=w59:bool)
      }
      frame #2 {
        n37 = local read "Timings"() -> (w74:dbl[][])
        n38 = Tick Count (ms)() -> (millisecond timer value=w77:u32)
        n39 = call "Timer.vi"("index"=3, "Timings in"=w74, "t1"=w78, "t2"=w77) -> ("Timings out"=w75:dbl[][])  [unwired: 2 in]
        n40 = Wait (ms)(milliseconds to wait="temp file interval (ms)") -> ()  [unwired: 1 out]
        n41 = local write "Timings"(w75) -> ()
      }
    }
  }
  n42 = while {
    tunnel: w1 -> [w84]
    shift-right: [w83] -> _
    shift-left: u64 0 -> [w81]
    tunnel: w4 -> [w80]
    stop <- w82 stop-if-true
    n43 = stacked-sequence {
      seq-local: [w85 _ _] -> [_ _ w207]
      tunnel: w84 -> [_ w104 _]
      tunnel: [_ w101 _] -> w83
      tunnel: [_ w98 _] -> w82
      tunnel: w81 -> [_ w90 _]
      tunnel: w80 -> [_ w86 _]
      frame #0 {
        n44 = Tick Count (ms)() -> (millisecond timer value=w85:u32)
      }
      frame #1 {
        # "Get sweep variable loop"
        n45 = Decrement(x=w90) -> (x-1=w91:u64)
        n46 = local read "start read vals"() -> (w92:bool)
        n47 = local read "Exp_params"() -> (w95:T15)
        n48 = Unbundle By Name(w95) -> ("sweep_dim"=w88:u64[])
        n49 = call "Count2Indexes.vi"("sweep_dim"=w88, "Count"=w91) -> ("Indexes"=w87:u64[])
        "Var index" <- w87
        n50 = Get Queue Status(queue=w104) -> (queue out=w100:refnum<queue>, # elements in queue=w103:i32)  [unwired: 2 in, 6 out]
        n51 = call "Count2Indexes.vi"("sweep_dim"=w88, "Count"=w90) -> ("Indexes"=w89:u64[])
        n52 = Less?(x=w103, y="Buf size") -> (x < y?=w93:bool)
        n53 = Decrement(x=w88) -> (x-1=w97:u64[])
        n54 = Equal?(x=w87, y=w97) -> (x = y?=w96:bool)
        n55 = And(x=w92, y=w93) -> (x .and. y?=w94:bool)
        n56 = case shown="True" w94 {
          tunnel: w88 -> [_ w118]
          tunnel: w90 -> [w105 w116]
          tunnel: [w105 w111] -> w101
          tunnel: w100 -> [_ w113]
          tunnel: w89 -> [_ w112]
          tunnel: w95 -> [_ w109]
          tunnel: w86 -> [_ w106]
          frame False {
          }
          frame True {
            w117 = 0
            n57 = Unbundle By Name(w109) -> ("sweep_list"=w108:string[])
            n58 = local read "Sweep inst info"() -> (w110:T12)
            n59 = Array Size(array=w118) -> (size(s)=w121:i32)
            n60 = Index Array(array=w118, index=w117) -> (element=w107:u64)
            n61 = Initialize Array(u32 1, w121) -> (w120:u32[])
            n62 = Add(x=w116, y=w107) -> (x+y=w111:u64)
            n63 = Replace Array Subset(array=w120, new element=w107, index=w117) -> (w115:u32[])
            n64 = for {
              shift-right: [w129] -> w114
              shift-left: cluster{string, "data":u16, dbl}[][] [] -> [w130]
              tunnel: w108 -> [w125] mode=indexing
              tunnel: w115 -> [w131]
              tunnel: w112 -> [w132]
              tunnel: w110 -> [w136] mode=indexing
              tunnel: w107 -> [w128]
              tunnel: w106 -> [w126]
              i -> [w127]
              n65 = Unbundle By Name(w136) -> ("Kind"=w135:u16)
              n66 = Not Equal?(x=11, y=w135) -> (x != y?=w133:bool)
              n67 = case shown="True" w133 {
                tunnel: w132 -> [_ w164]
                tunnel: w131 -> [_ w161]
                tunnel: w125 -> [_ w143]
                tunnel: w130 -> [w142 w155]
                tunnel: [w141 w154] -> w129
                tunnel: w128 -> [w139 _]
                tunnel: w127 -> [w137 w151]
                tunnel: w126 -> [_ w149]
                frame False {
                  # "Dummy points are created\nfor \"CMD\""
                  n68 = Initialize Array(cluster{string, "data":u64, dbl} {"None", "data"=100, 0.0}, w139) -> (w138:cluster{string, "data":u64, dbl}[])
                  n69 = Insert Into Array(array=w142, index (col)=w137, new element=w138) -> (w141:cluster{string, "data":u16, dbl}[][])  [unwired: 1 in]
                }
                frame True {
                  n70 = call <vilib>:"H5Fopen.vi"("mode (read-only)"=H5Fmode."read-only" ("mode"), "path"=w149) -> ("error out"=w144:errorcluster, "ref out"=w148:T13)  [unwired: 8 in]
                  n71 = call <vilib>:"H5Dget_space.vi"("error in (no error)"=w144, "obj (.)"=w143, "ref in"=w148) -> ("error out"=w168:errorcluster, "space out"=w162:T13)  [unwired: 7 in]
                  n72 = call <vilib>:"H5Sselect_simple.vi"("error in (no error)"=w168, "count"=w161, "start"=w164, "space in"=w162) -> ("error out"=w167:errorcluster, "space out"=w163:T13)  [unwired: 6 in]
                  n73 = xnode "H5Dread.xnode"("dataset name (this)"=w143, "error in (no error)"=w167, "default"=dbl[] [], "file space"=w163, "ref in"=w148) -> ("error out"=w166:errorcluster, "data"=w160:dbl[], "ref out"=w157:T13)  [unwired: 1 in, 1 out]
                  n74 = call <vilib>:"H5Sclose.vi"("error in (no error)"=w166, "space in"=w162) -> ("error out"=w147:errorcluster)  [unwired: 9 in]
                  n75 = xnode "H5Aread.xnode"("object name"=w143, "error in (no error)"=w147, "default"=u16 0, "attrib name"="parameter", "ref in"=w157) -> ("error out"=w146:errorcluster, "data"=w156:u16, "ref out"=w145:T13)  [unwired: 1 in, 1 out]
                  n76 = To Unsigned Quad Integer(1:w156) -> (0:w152:u64)
                  n77 = for {
                    tunnel: w160 -> [w187] mode=indexing
                    tunnel: w152 -> [w186]
                    tunnel: [w185] -> w153 mode=indexing
                    tunnel: w143 -> [w184]
                    n78 = Bundle(w184, w186, w187) -> (w185:cluster{string, u64, dbl})  [unwired: 1 in]
                  }
                  n79 = Insert Into Array(array=w155, index (col)=w151, new element=w153) -> (w154:cluster{string, "data":u16, dbl}[][])  [unwired: 1 in]
                  n80 = call <vilib>:"H5Fclose.vi"("error in (no error)"=w146, "ref"=w145) -> ()  [unwired: 9 in, 1 out]
                }
              }
            }
            n81 = for {
              tunnel: w114 -> [w124] mode=indexing
              tunnel: w113 -> [w123]
              n82 = Enqueue Element(queue=w123, element=w124) -> ()  [unwired: 2 in, 3 out]
            }
          }
        }
        n83 = local read "Stop"() -> (w99:bool)
        n84 = Or(x=w99, y=w96) -> (x .or. y?=w98:bool)
      }
      frame #2 {
        n85 = local read "Timings"() -> (w203:dbl[][])
        n86 = Tick Count (ms)() -> (millisecond timer value=w206:u32)
        n87 = call "Timer.vi"("index"=1, "Timings in"=w203, "t1"=w207, "t2"=w206) -> ("Timings out"=w204:dbl[][])  [unwired: 2 in]
        n88 = local write "Timings"(w204) -> ()
        n89 = Wait (ms)(milliseconds to wait="get variable interval (ms)") -> ()  [unwired: 1 out]
      }
    }
  }
  n90 = stacked-sequence {
    seq-local: [w209 _ _ _ _] -> [_ _ w332 _ _]
    tunnel: w7 -> [_ _ _ _ _]
    tunnel: [_ _ _ _ w856] -> w9
    tunnel: w1 -> [_ _ w336 _ _]
    tunnel: w5 -> [w210 _ _ _ _]
    tunnel: w3 -> [_ _ w335 w831 _]
    tunnel: w2 -> [_ _ w334 _ _]
    frame #0 {
      # "Initialize instruments and collect informations"
      # "Load experiment file"
      n91 = Tick Count (ms)() -> (millisecond timer value=w209:u32)
      n92 = Unbundle By Name(w210) -> ("Inst_parameters.Inst_array"=w218:T12, "Read out instrument bools"=w217:u64[][], "sweep_list"=w215:string[], "Sweep instrument bools"=w214:u64[][])
      n93 = Index Array(array=w214, index (col)=0) -> (element=w213:u64[])  [unwired: 1 in]
      n94 = Index Array(array=w217, index (col)=0) -> (element=w216:u64[])  [unwired: 1 in]
      n95 = call "Insts_init.vi"("Initialize sweep instruments ??"=w213, "sweep_list"=w215, "Initialize readout instruments??"=w216, "Inst_array"=w218) -> ("Sweep inst parameters"=→"Sweep inst info":T19, "Readout inst parameters"=→"Readout parameters":T19)
    }
    frame #1 {
      w223 = 0
      w222 = FALSE
      n96 = local write "start read vals"(TRUE) -> ()
      n97 = local read "Exp_params"() -> (w230:T15)
      n98 = Unbundle By Name(w230) -> ("Experimental bool list"=w235:bool[], "Inst_parameters.Inst_array"=w229:T12, "Sweep instrument bools"=w225:u64[][])
      n99 = Index Array(array=w225, index (col)=w223) -> (element=w224:u64[])  [unwired: 1 in]
      n100 = for {
        tunnel: w229 -> [w260] mode=indexing
        shift-right: [w262] -> w231
        shift-left: w222 -> [w263]
        shift-right: [w259] -> w236
        shift-left: "" -> [w261]
        shift-right: [w257] -> w228
        shift-left: w222 -> [w258]
        tunnel: w224 -> [w256]
        shift-right: [w253] -> _
        shift-left: w223 -> [w254]
        shift-right: [w251] -> w221
        shift-left: w222 -> [w252]
        # "Check DAC is used or not"
        n101 = Unbundle By Name(w260) -> ("Kind"=w255:u16)
        n102 = case shown="10" w255 {
          tunnel: w263 -> [w268 w273 w278 w283 _ _ _ _ w325 w329]
          tunnel: [w268 w273 w278 w283 TRUE w298 TRUE TRUE w325 w329] -> w262
          tunnel: w261 -> [w267 w272 w277 w282 _ _ _ _ w324 w330]
          tunnel: w260 -> [_ _ _ _ w291 w302 w310 w319 _ _]
          tunnel: [w267 w272 w277 w282 w288 w299 w307 w316 w324 w330] -> w259
          tunnel: w258 -> [w266 w271 w276 w281 w287 _ w306 w315 w323 w331]
          tunnel: [w266 w271 w276 w281 w287 w298 w306 w315 w323 w331] -> w257
          tunnel: w256 -> [_ _ _ _ _ w296 _ _ _ _]
          tunnel: w254 -> [w265 w270 w275 w280 w286 w295 w304 w314 w322 w327]
          tunnel: [w265 w270 w275 w280 w285 w297 w305 w313 w322 w328] -> w253
          tunnel: [w264 w269 w274 w279 w284 w293 w303 w312 w321 w326] -> w251
          tunnel: w252 -> [w264 w269 w274 w279 w284 _ w303 w312 w321 w326]
          frame 0 {
          }
          frame 1 {
          }
          frame 2 {
          }
          frame 3 {
          }
          frame 4 {
            # "DAC"
            n103 = Unbundle By Name(w291) -> ("Strings"=w290:string[])
            n104 = Index Array(array=w290, index=1) -> (element=w288:string)
            n105 = Increment(x=w286) -> (x+1=w285:i32)
          }
          frame 5 {
            w298 = TRUE
            # "DAC lock-in"
            n106 = Unbundle By Name(w302) -> ("Strings"=w301:string[])
            n107 = Index Array(array=w296, index=w295) -> (element=w294:u64)
            n108 = Index Array(array=w301, index=1) -> (element=w299:string)
            n109 = Not Equal To 0?(x=w294) -> (x != 0?=w293:bool)
            n110 = Increment(x=w295) -> (x+1=w297:i32)
            "DAC_lock-in_info" <- w302
          }
          frame 9 {
            # "Fast sequence"
            n111 = Unbundle By Name(w310) -> ("Strings"=w309:string[])
            n112 = Index Array(array=w309, index=1) -> (element=w307:string)
            n113 = Increment(x=w304) -> (x+1=w305:i32)
          }
          frame 10 {
            # "Fast sequence slot"
            n114 = Unbundle By Name(w319) -> ("Strings"=w318:string[])
            n115 = Index Array(array=w318, index=1) -> (element=w316:string)
            n116 = Increment(x=w314) -> (x+1=w313:i32)
          }
          frame 12 {
            # "DSP lock-in readout"
          }
          frame 100, Default {
            n117 = Increment(x=w327) -> (x+1=w328:i32)
          }
        }
      }
      n118 = Replace Array Subset(array=w235, new element=w231, index=1) -> (w233:bool[])
      n119 = Bundle By Name(cluster=w230, "Experimental bool list"=w233) -> (w232:T15)
      n120 = case shown="True" w231 {
        tunnel: w236 -> [_ w250]
        tunnel: w232 -> [w244 w249]
        tunnel: [w244 w248] -> w227
        tunnel: w229 -> [_ w245]
        frame False {
        }
        frame True {
          # "Initialize used busses"
          # "Get FPGA reference if DAC is used."
          # "Open FPGA"
          n121 = call "OpenFPGARef.vi"("IP Address"=w250) -> ("FPGA VI Reference Out"=w247:T14)
          n122 = call "DAC_set_use_buses.vi"("FPGA Ref"=w247, "Use FPGA?"=TRUE, "Inst_array"=w245) -> ()  [unwired: 1 out]
          n123 = Bundle By Name(cluster=w249, "FPGA Ref"=w247) -> (w248:T15)
        }
      }
      n124 = case shown="True" w228 {
        tunnel: w227 -> [_ w241]
        tunnel: w221 -> [_ w238]
        frame False {
        }
        frame True {
          # "DAC lock in init"
          n125 = local read "DAC_lock-in_info"() -> (w239:T4)
          n126 = Unbundle By Name(w241) -> ("FPGA Ref"=w240:T14)
          n127 = case shown="True" w238 {
            tunnel: w240 -> [_ w243]
            tunnel: w239 -> [_ w242]
            frame False {
            }
            frame True {
              # "check sweep inst\nbool"
              n128 = call "DAC_lock_in_init.vi"("Inst info"=w242, "FPGA VI Reference In"=w243) -> ()  [unwired: 1 in]
            }
          }
        }
      }
      n129 = local write "Exp_params"(w227) -> ()
    }
    frame #2 {
      # "Check mode"
      n130 = local read "Exp_params"() -> (w339:T15)
      n131 = Unbundle By Name(w339) -> ("Inst_parameters.fast_mode"=w338:u8[])
      n132 = call "Sweep_mode.vi"("fast_mode"=w338) -> ("ramp?"=w337:bool, "Sweep mode"=w333:enum16{"Normal sweep", "Fast sweep"})  [unwired: 1 in]
      n133 = case shown="\"Fast sweep\"" w333 {
        tunnel: u64 0 -> [w360 w541]
        tunnel: w339 -> [w356 w531]
        tunnel: w337 -> [_ w533]
        tunnel: w334 -> [w347 w529]
        tunnel: w336 -> [w346 w528]
        tunnel: w335 -> [w343 w525]
        tunnel: w332 -> [w341 w523]
        frame "Normal sweep", Default {
          n134 = Unbundle By Name(w356) -> ("Initial move"=w345:T3, "sweep_dim"=w355:u64[], "ExpFilePath"=w342:path, "sweep_list"=w354:string[], "Inst_parameters.Wait_times"=w353:u64[], "readout_list"=w352:string[], "FPGA Ref"=w350:T14, "Experimental bool list"=w349:bool[], "Inst_parameters.Inst_array"=w344:T12)
          n135 = local read "Readout parameters"() -> (w358:T12)
          n136 = local read "Sweep inst info"() -> (w357:T12)
          n137 = Index Array(array=w349, index=1) -> (element=w348:bool)
          n138 = stacked-sequence {
            seq-local: [w361 _ _] -> [_ w382 _]
            seq-local: [_ w383 _] -> [_ _ w399]
            tunnel: w360 -> [_ _ w416]
            tunnel: 0 -> [_ _ w415]
            tunnel: w358 -> [_ _ w414]
            tunnel: w357 -> [_ _ w413]
            tunnel: w355 -> [w372 _ w412]
            tunnel: w354 -> [_ _ w411]
            tunnel: w353 -> [w370 _ w410]
            tunnel: w352 -> [_ _ w409]
            tunnel: w350 -> [w369 w390 w408]
            tunnel: w348 -> [w367 w389 w407]
            tunnel: w347 -> [_ _ w406]
            tunnel: w346 -> [_ _ w405]
            tunnel: w345 -> [w371 _ _]
            tunnel: w344 -> [w368 w391 _]
            tunnel: w343 -> [w366 _ w404]
            tunnel: w342 -> [_ w388 _]
            tunnel: w341 -> [w362 _ _]
            frame #0 {
              # "Perform initial movement"
              # "Collect information of the instruments\nto be moved at the beggining."
              # "Wait after initial movement"
              n139 = local read "Timings"() -> (w364:dbl[][])
              n140 = Tick Count (ms)() -> (millisecond timer value=w361:u32)
              n141 = call "Timer.vi"("index"=4, "Timings in"=w364, "t1"=w362, "t2"=w361) -> ("Timings out"=w365:dbl[][])  [unwired: 2 in]
              n142 = Index Array(array=w370, index=0) -> (element=w374:u64)
              n143 = local write "Timings"(w365) -> ()
              n144 = call "Select_inst_info.vi"("Inst_parameters.Inst_array"=w368, "Initial move"=w371) -> ("Inst_parameters.Inst_array 2"=w373:T12)
              n145 = flat-sequence {
                tunnel: w371 -> [w378]
                tunnel: w369 -> [w380]
                tunnel: w373 -> [w379]
                tunnel: w367 -> [w377]
                tunnel: w366 -> [w376]
                tunnel: w374 -> [w381]
                frame #0 {
                  # "Move"
                  n146 = call "Move.vi"("Points"=w378, "Sweep inst info"=w379, "FPGA Ref"=w380, "Use FPGA?"=w377, "WorkFilePath"=w376) -> ()  [unwired: 5 in, 1 out]
                }
                frame #1 {
                  # "Initial wait (ms)"
                  n147 = Wait (ms)(milliseconds to wait=w381) -> ()  [unwired: 1 out]
                }
              }
              "sweep_dim" <- w372
            }
            frame #1 {
              # "Register value of all the instruments before the measurement"
              n148 = local read "Timings"() -> (w385:dbl[][])
              n149 = Tick Count (ms)() -> (millisecond timer value=w383:u32)
              n150 = call "Timer.vi"("index"=7, "Timings in"=w385, "t1"=w382) -> ("Timings out"=w386:dbl[][])  [unwired: 3 in]
              n151 = local write "Timings"(w386) -> ()
              n152 = call "GetTempFilePath.vi"("ExpFilePath"=w388) -> ("Temp file path"=w387:path)
              n153 = case shown="True" w389 {
                tunnel: w390 -> [_ w398]
                tunnel: [w394 w397] -> w392
                frame False {
                  w396 = 8
                  n154 = Initialize Array(0.0, w396, w396) -> (w394:dbl[][])
                }
                frame True {
                  n155 = call "DAC_current_values.vi"("FPGA Ref"=w398) -> ("DAC values"=w397:sgl[][])
                }
              }
              n156 = call "Get_values.vi"("DAC values"=w392, "Inst_array"=w391, "Temp file path"=w387) -> ("Initial positions"=→"Initial positions":T3)
            }
            frame #2 {
              n157 = while {
                shift-right: [w442] -> _
                shift-left: w416 -> [w428]
                shift-right: [w436] -> _
                shift-left: w415 -> [w437]
                tunnel: w414 -> [w434]
                tunnel: w413 -> [w427]
                tunnel: w412 -> [w433]
                tunnel: w411 -> [w422]
                tunnel: w410 -> [w432]
                tunnel: w409 -> [w431]
                tunnel: w408 -> [w430]
                tunnel: w407 -> [w429]
                tunnel: w406 -> [w426]
                tunnel: w405 -> [w425]
                tunnel: w404 -> [w420]
                stop <- w441 stop-if-true
                # "Seep indexes"
                # "Stop if stop button is pushed or\nindex reaches the sweep dimension."
                n158 = Array Size(array=w422) -> (size(s)=w423:i32)
                n159 = Not Equal To 0?(x=w423) -> (x != 0?=w421:bool)
                n160 = case shown="True" w421 {
                  tunnel: w425 -> [_ w445]
                  tunnel: [cluster{string, "data":u64, dbl}[] [{"None", "data"=100, 0.0}] w444] -> w424
                  frame False {
                  }
                  frame True {
                    n161 = Dequeue Element(queue=w445) -> (element=w444:cluster{string, "data":u64, dbl}[])  [unwired: 2 in, 3 out]
                  }
                }
                n162 = call "Count2Indexes.vi"("sweep_dim"=w433, "Count"=w428) -> ("Indexes"=w439:u64[])
                "Indexes" <- w439
                n163 = Tick Count (ms)() -> (millisecond timer value=w418:u32)
                n164 = stacked-sequence {
                  seq-local: [_ _ _ w480 _ _ _] -> [_ _ _ _ w492 w497 _]
                  seq-local: [_ _ w455 _ _ _ _] -> [_ _ _ _ w486 _ _]
                  seq-local: [_ _ _ _ w485 _ _] -> [_ _ _ _ _ _ w518]
                  tunnel: w427 -> [w449 _ _ _ _ _ _]
                  tunnel: w432 -> [_ w454 w460 w483 _ _ _]
                  tunnel: w434 -> [_ _ _ w481 _ _ _]
                  tunnel: w439 -> [w448 _ w463 _ _ w493 w522]
                  tunnel: w433 -> [_ _ _ _ _ w498 w511]
                  tunnel: w431 -> [_ _ _ _ _ _ _]
                  tunnel: [_ _ _ _ _ _ w511] -> w419
                  tunnel: [_ _ _ _ _ _ w522] -> w417
                  tunnel: w437 -> [_ _ w462 _ _ _ _]
                  tunnel: [_ _ w461 _ _ _ _] -> w436
                  tunnel: w430 -> [w451 _ _ _ _ _ _]
                  tunnel: w429 -> [w450 _ _ _ _ _ _]
                  tunnel: w428 -> [_ _ _ _ _ _ w510]
                  tunnel: w426 -> [_ _ _ _ w487 _ _]
                  tunnel: w424 -> [w446 _ _ _ _ w495 _]
                  tunnel: w420 -> [w447 _ _ _ _ _ _]
                  tunnel: w418 -> [_ _ w456 _ _ _ w514]
                  frame #0 {
                    # "Move to the position"
                    n165 = call "Move.vi"("Points"=w446, "Sweep inst info"=w449, "FPGA Ref"=w451, "Use FPGA?"=w450, "WorkFilePath"=w447, "Indexes"=w448) -> ()  [unwired: 4 in, 1 out]
                  }
                  frame #1 {
                    # "Wait before measurement"
                    n166 = Index Array(array=w454, index=1) -> (element=w452:u64)
                    n167 = Wait (ms)(milliseconds to wait=w452) -> ()  [unwired: 1 out]
                  }
                  frame #2 {
                    # "Extra wait time\nwhen we step."
                    # "Wait after step movement"
                    n168 = Array Size(array=w463) -> (size(s)=w465:i32)
                    n169 = Tick Count (ms)() -> (millisecond timer value=w455:u32)
                    n170 = Greater?(x=w465, y=1) -> (0:w466:bool)
                    n171 = case shown="True" w466 {
                      tunnel: w463 -> [_ w474]
                      tunnel: w462 -> [w467 w471]
                      tunnel: [w467 w470] -> w461
                      tunnel: w460 -> [_ w468]
                      frame False {
                      }
                      frame True {
                        n172 = Index Array(array=w474, index=1) -> (element=w469:u64)
                        n173 = Equal?(x=w469, y=w471) -> (x = y?=w472:bool)
                        n174 = case shown="False" w472 {
                          tunnel: w471 -> [_ w479]
                          tunnel: [w478 w479] -> w470
                          tunnel: w469 -> [w478 _]
                          tunnel: w468 -> [w477 _]
                          frame False {
                            n175 = Index Array(array=w477, index=3) -> (element=w475:u64)
                            n176 = Wait (ms)(milliseconds to wait=w475) -> ()  [unwired: 1 out]
                          }
                          frame True {
                          }
                        }
                      }
                    }
                    n177 = local read "Timings"() -> (w458:dbl[][])
                    n178 = call "Timer.vi"("index"=10, "Timings in"=w458, "t1"=w456, "t2"=w455) -> ("Timings out"=w457:dbl[][])  [unwired: 2 in]
                    n179 = local write "Timings"(w457) -> ()
                  }
                  frame #3 {
                    # "Readout data"
                    n180 = Index Array(array=w483, index=2) -> (element=w482:u64)
                    n181 = call "Read.vi"("Readout parameters"=w481, "Integration time (ms)"=w482) -> ("Data"=w480:dbl[])  [unwired: 1 in]
                  }
                  frame #4 {
                    # "Save data to the file"
                    n182 = Build Array(w492) -> (w491:dbl[][])
                    n183 = local write "Temp data"(w491) -> ()
                    n184 = Enqueue Element(queue=w487, element=w491) -> ()  [unwired: 2 in, 3 out]
                    n185 = local read "Timings"() -> (w489:dbl[][])
                    n186 = Tick Count (ms)() -> (millisecond timer value=w485:u32)
                    n187 = call "Timer.vi"("index"=14, "Timings in"=w489, "t1"=w486, "t2"=w485) -> ("Timings out"=w488:dbl[][])  [unwired: 2 in]
                    n188 = local write "Timings"(w488) -> ()
                  }
                  frame #5 {
                    n189 = local read "Plot parameters"() -> (w494:T2)
                    n190 = Unbundle By Name(w494) -> ("Disable plot"=w496:bool)
                    n191 = case shown="False" w496 {
                      tunnel: w498 -> [w504 _]
                      tunnel: w497 -> [w502 _]
                      tunnel: w495 -> [w508 _]
                      tunnel: w493 -> [w505 _]
                      frame False {
                        # "Add data to plot queue"
                        n192 = local read "Plot parameters"() -> (w506:T2)
                        n193 = Build Array(w502) -> (w499:dbl[][])
                        n194 = Array Size(array=w502) -> (size(s)=w501:i32)
                        n195 = Array Size(array=w499) -> (size(s)=w500:i32[])
                        n196 = Index Array(array=w499, index (row)=w501) -> ()  [unwired: 1 in, 1 out]
                        n197 = Index Array(array=w500) -> ()  [unwired: 1 in, 1 out]
                        n198 = call "Plot_add_to_buffer.vi"("Plot parameters in"=w506, "fast mode"=enum16{"normal sweep", "fast sweep"}."normal sweep", "Points"=w508, "new_data"=w499, "sweep_dim"=w504, "Indexes"=w505) -> ("Plot parameters out"=w507:T2)  [unwired: 1 in]
                        n199 = local write "Plot parameters"(w507) -> ()
                      }
                      frame True {
                      }
                    }
                  }
                  frame #6 {
                    # "Sweep counter check"
                    n200 = local read "Timings"() -> (w516:dbl[][])
                    n201 = local read "Timings"() -> (w520:dbl[][])
                    n202 = Tick Count (ms)() -> (millisecond timer value=w517:u32)
                    n203 = Tick Count (ms)() -> (millisecond timer value=w519:u32)
                    n204 = call "Timer.vi"("index"=9, "Timings in"=w516, "t1"=w514, "t2"=w517) -> ("Timings out"=w512:dbl[][])  [unwired: 2 in]
                    n205 = call "Timer.vi"("index"=2, "Timings in"=w520, "t1"=w518, "t2"=w519) -> ("Timings out"=w513:dbl[][])  [unwired: 2 in]
                    n206 = local write "Timings"(w512) -> ()
                    n207 = local write "Timings"(w513) -> ()
                    n208 = call "RemainingTime.vi"("Timings"=w512, "sweep_dim"=w511, "Count"=w510) -> ("Remaning time (min)"=w509:dbl)
                    n209 = local write "Remaning time (min)"(w509) -> ()
                  }
                }
                n210 = Decrement(x=w419) -> (x-1=w435:u64[])
                n211 = Equal?(x=w417, y=w435) -> (x = y?=w438:bool)
                n212 = local read "Stop"() -> (w440:bool)
                n213 = Increment(x=w428) -> (x+1=w442:u64)
                n214 = Or(x=w438, y=w440) -> (x .or. y?=w441:bool)
              }
              n215 = local read "Timings"() -> (w401:dbl[][])
              n216 = Tick Count (ms)() -> (millisecond timer value=w403:u32)
              n217 = call "Timer.vi"("index"=6, "Timings in"=w401, "t1"=w399, "t2"=w403) -> ("Timings out"=w400:dbl[][])  [unwired: 2 in]
              n218 = local write "Timings"(w400) -> ()
            }
          }
        }
        frame "Fast sweep" {
          (unwired) 0
          # "Number of points to keep"
          # "File ref"
          # "Type of reding instrument\nex.) ADC, K2000, Lecroy\n(We asuume that we only\nuse 1 kind of an instrument\nat a time. If this condition is\nnot met, error comes out.)"
          # "Number of point to acquire"
          # "FPGA ref"
          n219 = Unbundle By Name(w531) -> ("Initial move"=w527:T3, "FPGA Ref"=w532:T14, "Inst_parameters.ConfigFilePath"=w534:path, "sweep_dim"=w535:u64[], "sweep_list"=w538:string[], "readout_list"=w537:string[], "Inst_parameters.Wait_times"=w536:u64[], "Experimental bool list"=w530:bool[], "Inst_parameters.Inst_array"=w526:T12, "ExpFilePath"=w524:path)
          n220 = local read "Sweep inst info"() -> (w539:T12)
          n221 = local read "Readout parameters"() -> (w540:T12)
          n222 = stacked-sequence {
            seq-local: [_ w572 _ _ _ _ _] -> [_ _ w590 _ _ w669 _]
            seq-local: [w544 _ _ _ _ _ _] -> [_ w571 w588 _ _ w673 w822]
            seq-local: [_ w565 _ _ _ _ _] -> [_ _ _ _ _ w668 _]
            seq-local: [_ w560 _ _ _ _ _] -> [_ _ w582 _ _ _ _]
            seq-local: [_ _ w583 _ _ _ _] -> [_ _ _ w621 _ _ _]
            seq-local: [_ _ _ w622 _ _ _] -> [_ _ _ _ w644 _ _]
            seq-local: [_ _ _ _ w645 _ _] -> [_ _ _ _ _ w663 _]
            tunnel: w541 -> [_ _ _ _ _ w681 _]
            tunnel: w540 -> [_ _ w587 _ _ _ _]
            tunnel: w539 -> [_ _ _ _ _ w678 _]
            tunnel: w538 -> [_ _ _ _ _ w679 _]
            tunnel: w537 -> [_ _ _ _ _ w675 _]
            tunnel: w536 -> [_ _ _ w634 _ w677 _]
            tunnel: w535 -> [_ _ _ w627 _ w680 _]
            tunnel: w534 -> [w550 _ _ _ _ _ _]
            tunnel: w533 -> [_ w570 w589 _ _ w676 _]
            tunnel: w532 -> [w545 _ _ w630 w654 _ _]
            tunnel: w531 -> [w549 _ _ _ _ _ _]
            tunnel: w530 -> [w547 _ _ w632 w653 w674 _]
            tunnel: w529 -> [_ _ _ _ _ w672 _]
            tunnel: w528 -> [_ _ _ _ _ w671 _]
            tunnel: w527 -> [_ _ _ w629 _ _ _]
            tunnel: w526 -> [_ _ _ w628 w652 _ _]
            tunnel: w525 -> [_ _ _ w626 _ w670 _]
            tunnel: w524 -> [_ _ _ _ w651 _ _]
            tunnel: w523 -> [_ w561 _ _ _ _ _]
            frame #0 {
              # "Get fast sequence inforamtion"
              n223 = call "Get_fast_seq_info.vi"("ConfigFilePath"=w550) -> ("Fast sequence parameters"=w543:T11)
              "Fast sequence parameters" <- w543
              n224 = Unbundle By Name(w543) -> ("IP address"=w542:string)
              n225 = Index Array(array=w547, index=1) -> (element=w546:bool)
              n226 = case shown="False" w546 {
                tunnel: w549 -> [w558 _]
                tunnel: w547 -> [w557 _]
                tunnel: w545 -> [_ w559]
                tunnel: [w552 w559] -> w544
                tunnel: w542 -> [w551 _]
                frame False {
                  # "Update use FPGA status here if it is FALSE before"
                  n227 = call "OpenFPGARef.vi"("IP Address"=w551) -> ("FPGA VI Reference Out"=w552:T14)
                  n228 = Replace Array Subset(array=w557, new element=TRUE, index=1) -> (w554:bool[])
                  n229 = Bundle By Name(cluster=w558, "Experimental bool list"=w554, "FPGA Ref"=w552) -> (w553:T15)
                  n230 = local write "Exp_params"(w553) -> ()
                }
                frame True {
                }
              }
            }
            frame #1 {
              # "Initialize the fast sequence"
              n231 = local read "Timings"() -> (w562:dbl[][])
              n232 = local read "Fast sequence parameters"() -> (w569:T11)
              n233 = call "Fast_seq_init.vi"("FPGA Ref"=w571, "Ramp?"=w570, "Fast sequence parameters 2"=w569) -> ()
              n234 = Tick Count (ms)() -> (millisecond timer value=w560:u32)
              n235 = Unbundle By Name(w569) -> ("Sequence size"=w574:u64, "Sample count"=w573:u64, "Start ramp at"=w566:u64, "fastseq"=w568:T20, "Fast-seq-divider"=w567:u64)
              n236 = call "Timer.vi"("index"=4, "Timings in"=w562, "t1"=w561, "t2"=w560) -> ("Timings out"=w563:dbl[][])  [unwired: 2 in]
              n237 = local write "Timings"(w563) -> ()
              n238 = case shown="True" w570 {
                tunnel: [w575 w577] -> w572
                tunnel: w574 -> [_ w578]
                tunnel: w573 -> [w575 _]
                tunnel: w568 -> [_ w581]
                tunnel: w567 -> [_ w580]
                tunnel: w566 -> [_ w579]
                tunnel: [w575 w576] -> w565
                frame False {
                }
                frame True {
                  n239 = call "Convert_pre_ramp_sequence.vi"("Fast-seq-divider"=w580, "fastseq"=w581, "Start ramp at"=w579, "Sequence size"=w578) -> ("Pts to acquire"=w577:u64, "Pts to keep"=w576:u64)
                }
              }
            }
            frame #2 {
              # "Configure and initialize voltmeters for fast ramp"
              n240 = local read "Timings"() -> (w585:dbl[][])
              n241 = Tick Count (ms)() -> (millisecond timer value=w583:u32)
              n242 = call "Timer.vi"("index"=5, "Timings in"=w585, "t1"=w582, "t2"=w583) -> ("Timings out"=w586:dbl[][])  [unwired: 2 in]
              n243 = local write "Timings"(w586) -> ()
              n244 = for {
                tunnel: w587 -> [w596] mode=indexing
                tunnel: w590 -> [w595]
                tunnel: w589 -> [w594]
                tunnel: w588 -> [w593]
                tunnel: w587 -> [w592]
                i -> [w591]
                n245 = Unbundle By Name(w596) -> ("Kind"=w597:u16)
                n246 = case shown="0" w597 {
                  tunnel: w596 -> [w600 w609 _ w619 _]
                  tunnel: w595 -> [w605 w608 _ w617 _]
                  tunnel: w594 -> [w606 _ _ w618 _]
                  tunnel: w593 -> [_ w607 _ w620 _]
                  tunnel: w592 -> [w602 _ _ _ _]
                  tunnel: w591 -> [w601 _ _ _ _]
                  frame 0 {
                    # "Update take out\nand sample per\nchannel"
                    # "ADC"
                    n247 = local read "Fast sequence parameters"() -> (w604:T11)
                    n248 = Unbundle By Name(w604) -> ("Fast-seq-divider"=w603:u64)
                    n249 = call "ADC_config_fastsweep.vi"("Inst_parameter"=w600, "Fast sequence size"=w605, "fast sequence divider"=w603, "Ramp?"=w606) -> ("Inst_parameter out"=w598:T4)  [unwired: 1 in]
                    n250 = Replace Array Subset(array=w602, new element=w598, index=w601) -> (w599:T12)
                    n251 = local write "Readout parameters"(w599) -> ()
                  }
                  frame 1 {
                    # "K2000"
                    n252 = stacked-sequence {
                      tunnel: w609 -> [w612 w616]
                      tunnel: w608 -> [w611 _]
                      tunnel: w607 -> [w610 _]
                      frame #0 {
                        n253 = call "K2000_config_fastsweep.vi"("Readout_inst_parameters"=w612, "readings"=w611) -> ()  [unwired: 1 in, 1 out]
                        n254 = call "DAC_set_stop-sample-count.vi"("FPGA VI Reference In"=w610) -> ()  [unwired: 1 in, 10 out]
                      }
                      frame #1 {
                        n255 = Unbundle By Name(w616) -> ("Strings"=w615:string[])
                        n256 = Index Array(array=w615, index=1) -> (element=w613:string)
                        n257 = call "K2000_init_fastseq.vi"("GPIB address"=w613) -> ()
                      }
                    }
                  }
                  frame 3 {
                    # "LeCroy"
                  }
                  frame 12 {
                    # "Lock-in"
                    n258 = call "DSP_init_fast_sweep.vi"("Sample count"=w617, "ramp?"=w618, "Inst info"=w619) -> ()  [unwired: 1 in]
                    n259 = call "DAC_set_stop-sample-count.vi"("FPGA VI Reference In"=w620) -> ()  [unwired: 1 in, 10 out]
                  }
                  frame 100, Default {
                  }
                }
              }
            }
            frame #3 {
              # "Perform initial movement"
              # "Collect information of the instruments\nto be moved at the beggining."
              # "Wait after initial movement"
              n260 = local write "sweep_dim"(w627) -> ()
              n261 = Index Array(array=w632, index=1) -> (element=w631:bool)
              n262 = local read "Timings"() -> (w624:dbl[][])
              n263 = Tick Count (ms)() -> (millisecond timer value=w622:u32)
              n264 = call "Timer.vi"("index"=6, "Timings in"=w624, "t1"=w621, "t2"=w622) -> ("Timings out"=w625:dbl[][])  [unwired: 2 in]
              n265 = local write "Timings"(w625) -> ()
              n266 = Index Array(array=w634, index=0) -> (element=w636:u64)
              n267 = call "Select_inst_info.vi"("Inst_parameters.Inst_array"=w628, "Initial move"=w629) -> ("Inst_parameters.Inst_array 2"=w635:T12)
              n268 = flat-sequence {
                tunnel: w629 -> [w640]
                tunnel: w630 -> [w642]
                tunnel: w635 -> [w641]
                tunnel: w631 -> [w639]
                tunnel: w626 -> [w638]
                tunnel: w636 -> [w643]
                frame #0 {
                  # "Move"
                  n269 = call "Move.vi"("Points"=w640, "Sweep inst info"=w641, "FPGA Ref"=w642, "Use FPGA?"=w639, "WorkFilePath"=w638) -> ()  [unwired: 5 in, 1 out]
                }
                frame #1 {
                  # "Initial wait (ms)"
                  n270 = Wait (ms)(milliseconds to wait=w643) -> ()  [unwired: 1 out]
                }
              }
            }
            frame #4 {
              # "Register value of all the instruments before the measurement"
              n271 = call "GetTempFilePath.vi"("ExpFilePath"=w651) -> ("Temp file path"=w650:path)
              n272 = local read "Timings"() -> (w647:dbl[][])
              n273 = Tick Count (ms)() -> (millisecond timer value=w645:u32)
              n274 = call "Timer.vi"("index"=7, "Timings in"=w647, "t1"=w644, "t2"=w645) -> ("Timings out"=w648:dbl[][])  [unwired: 2 in]
              n275 = local write "Timings"(w648) -> ()
              n276 = Index Array(array=w653, index=1) -> (element=w656:bool)
              n277 = case shown="True" w656 {
                tunnel: w654 -> [_ w662]
                tunnel: [w658 w661] -> w655
                frame False {
                  w660 = 8
                  n278 = Initialize Array(0.0, w660, w660) -> (w658:dbl[][])
                }
                frame True {
                  n279 = call "DAC_current_values.vi"("FPGA Ref"=w662) -> ("DAC values"=w661:sgl[][])
                }
              }
              n280 = call "Get_values.vi"("DAC values"=w655, "Inst_array"=w652, "Temp file path"=w650) -> ("Initial positions"=w649:T3)
              n281 = local write "Initial positions"(w649) -> ()
            }
            frame #5 {
              # "Measurement loop"
              n282 = while {
                shift-right: [w708] -> _
                shift-left: w681 -> [w695]
                tunnel: w680 -> [w705]
                tunnel: w679 -> [w688]
                tunnel: w678 -> [w694]
                tunnel: w677 -> [w703]
                tunnel: w676 -> [w702]
                tunnel: w669 -> [w701]
                tunnel: w675 -> [w700]
                tunnel: w674 -> [w698]
                tunnel: w673 -> [w697]
                tunnel: w672 -> [w693]
                tunnel: w671 -> [w692]
                tunnel: w670 -> [w687]
                tunnel: w668 -> [w685]
                tunnel: w669 -> [w684]
                stop <- w686 stop-if-true
                n283 = local read "Readout parameters"() -> (w696:T12)
                n284 = Array Size(array=w688) -> (size(s)=w690:i32)
                n285 = Not Equal To 0?(x=w690) -> (x != 0?=w689:bool)
                n286 = call "Count2Indexes.vi"("sweep_dim"=w705, "Count"=w695) -> ("Indexes"=w699:u64[])
                n287 = case shown="True" w689 {
                  tunnel: w692 -> [_ w711]
                  tunnel: [cluster{string, "data":u64, dbl}[] [{"None", "data"=100, 0.0}] w710] -> w691
                  frame False {
                  }
                  frame True {
                    n288 = Dequeue Element(queue=w711) -> (element=w710:cluster{string, "data":u64, dbl}[])  [unwired: 2 in, 3 out]
                  }
                }
                n289 = stacked-sequence {
                  seq-local: [_ _ w731 _ _ _ _ _ _] -> [_ _ _ w748 _ w768 _ _ _]
                  seq-local: [_ _ _ _ w750 _ _ _ _] -> [_ _ _ _ _ _ w777 w797 _]
                  seq-local: [_ _ w726 _ _ _ _ _ _] -> [_ _ _ w744 _ _ _ _ _]
                  seq-local: [_ _ _ w743 _ _ _ _ _] -> [_ _ _ _ w753 _ _ _ _]
                  seq-local: [_ _ _ _ w752 _ _ _ _] -> [_ _ _ _ _ w764 _ _ _]
                  seq-local: [_ _ _ _ _ w763 _ _ _] -> [_ _ _ _ _ _ w772 _ _]
                  seq-local: [_ _ _ _ _ _ w770 _ _] -> [_ _ _ _ _ _ _ w791 _]
                  seq-local: [_ _ _ _ _ _ _ w790 _] -> [_ _ _ _ _ _ _ _ w809]
                  seq-local: [w712 _ _ _ _ _ _ _ _] -> [_ _ w725 _ _ _ _ _ w808]
                  tunnel: w699 -> [w715 _ _ _ _ _ _ w799 w817]
                  tunnel: w705 -> [_ _ _ _ _ _ _ w798 w816]
                  tunnel: [_ _ _ _ _ _ _ _ w816] -> w683
                  tunnel: [_ _ _ _ _ _ _ _ w817] -> w704
                  tunnel: w694 -> [w716 _ _ _ _ _ _ _ _]
                  tunnel: w703 -> [_ w723 _ _ _ _ _ _ _]
                  tunnel: w702 -> [_ _ w733 _ _ _ w775 _ _]
                  tunnel: w701 -> [_ _ w732 _ w762 _ _ _ _]
                  tunnel: w696 -> [_ _ _ _ _ _ w778 _ _]
                  tunnel: w700 -> [_ _ _ _ _ _ _ _ _]
                  tunnel: w698 -> [w721 _ _ _ _ _ _ _ _]
                  tunnel: w697 -> [w718 _ w730 _ _ _ _ _ _]
                  tunnel: [w717 _ _ _ _ _ _ _ _] -> _
                  tunnel: w695 -> [_ _ _ _ _ _ _ _ w815]
                  tunnel: w693 -> [_ _ _ _ _ _ w776 _ _]
                  tunnel: w691 -> [w714 _ _ _ _ _ _ w796 _]
                  tunnel: w687 -> [w713 _ _ _ _ _ _ _ _]
                  tunnel: w685 -> [_ _ _ _ w758 _ _ _ _]
                  tunnel: w684 -> [_ _ _ _ w759 _ _ _ _]
                  frame #0 {
                    # "Move to the point"
                    n290 = Tick Count (ms)() -> (millisecond timer value=w712:u32)
                    n291 = Index Array(array=w721, index=1) -> (element=w720:bool)
                    n292 = call "Move.vi"("Points"=w714, "Sweep inst info"=w716, "FPGA Ref"=w718, "Use FPGA?"=w720, "WorkFilePath"=w713, "Indexes"=w715) -> ("FPGA VI Reference Out"=w717:T14)  [unwired: 4 in]
                  }
                  frame #1 {
                    # "Wait after step movement\n(For the fast sequence there is no wait\nbetween sweep measurement)"
                    n293 = Index Array(array=w723, index=3) -> (element=w722:u64)
                    n294 = Wait (ms)(milliseconds to wait=w722) -> ()  [unwired: 1 out]
                  }
                  frame #2 {
                    # "Start fast sequence at the new sweep"
                    n295 = local read "Timings"() -> (w728:dbl[][])
                    n296 = Tick Count (ms)() -> (millisecond timer value=w726:u32)
                    n297 = case shown="True" w733 {
                      tunnel: w732 -> [w736 w738]
                      tunnel: [w735 w740] -> w731
                      tunnel: w730 -> [w734 w741]
                      frame False {
                        n298 = call "DAC_set_stop-sample-count.vi"("sample count"=w736, "FPGA VI Reference In"=w734) -> ("FPGA VI Reference Out"=w735:T14)  [unwired: 9 out]
                      }
                      frame True {
                        n299 = Add(x=w738, y=0) -> (x+y=w739:u64)
                        n300 = call "fastseq_set_orders.vi"("FPGA VI Reference In"=w741, "sample count"=w739, "Enum"=T18."set ramp") -> ("FPGA VI Reference Out"=w740:T14)  [unwired: 2 in]
                      }
                    }
                    n301 = call "Timer.vi"("index"=10, "Timings in"=w728, "t1"=w725, "t2"=w726) -> ("Timings out"=w727:dbl[][])  [unwired: 2 in]
                    n302 = local write "Timings"(w727) -> ()
                  }
                  frame #3 {
                    # "Start fast sequence"
                    n303 = local read "Timings"() -> (w746:dbl[][])
                    n304 = Tick Count (ms)() -> (millisecond timer value=w743:u32)
                    n305 = call "Timer.vi"("index"=11, "Timings in"=w746, "t1"=w744, "t2"=w743) -> ("Timings out"=w745:dbl[][])  [unwired: 2 in]
                    n306 = call "fastseq_set_orders.vi"("FPGA VI Reference In"=w748, "Enum"=T18."start") -> ()  [unwired: 3 in, 1 out]
                    n307 = local write "Timings"(w745) -> ()
                  }
                  frame #4 {
                    # "Read data"
                    n308 = local read "Readout parameters"() -> (w761:T12)
                    n309 = Subtract(x=w759, y=w758) -> (x-y=w757:u64)
                    n310 = call "Read_fastseq.vi"("Sequence size"=w762, "Readout parameters"=w761) -> ("measures"=w751:sgl[][], "Readout parameters out"=w760:T12)  [unwired: 2 in]
                    n311 = local read "Timings"() -> (w755:dbl[][])
                    n312 = Array Subset(array=w751, index (col)=w757, length (col)=w758) -> (w750:sgl[][])  [unwired: 2 in]
                    "Temp data" <- w750
                    n313 = Tick Count (ms)() -> (millisecond timer value=w752:u32)
                    n314 = local write "Readout parameters"(w760) -> ()
                    n315 = call "Timer.vi"("index"=12, "Timings in"=w755, "t1"=w753, "t2"=w752) -> ("Timings out"=w754:dbl[][])  [unwired: 2 in]
                    n316 = local write "Timings"(w754) -> ()
                  }
                  frame #5 {
                    # "Stop fast sequence"
                    n317 = local read "Timings"() -> (w766:dbl[][])
                    n318 = call "fastseq_set_orders.vi"("FPGA VI Reference In"=w768, "Enum"=T18."stop") -> ()  [unwired: 3 in, 1 out]
                    n319 = Tick Count (ms)() -> (millisecond timer value=w763:u32)
                    n320 = call "Timer.vi"("index"=14, "Timings in"=w766, "t1"=w764, "t2"=w763) -> ("Timings out"=w765:dbl[][])  [unwired: 2 in]
                    n321 = local write "Timings"(w765) -> ()
                  }
                  frame #6 {
                    # "Save array data"
                    # "Clear buffer before going to next"
                    n322 = for {
                      tunnel: w778 -> [w782] mode=indexing
                      tunnel: w778 -> [w781]
                      tunnel: w775 -> [w779]
                      i -> [w780]
                      n323 = Unbundle By Name(w782) -> ("Kind"=w783:u16)
                      n324 = case shown="0" w783 {
                        tunnel: w782 -> [w787 w788 _]
                        tunnel: w781 -> [w786 _ _]
                        tunnel: w780 -> [w785 _ _]
                        tunnel: w779 -> [_ w789 _]
                        frame 0 {
                          n325 = call "ADC_clean_buffer_batch.vi"("Index"=w785, "Readout parameters in"=w786, "Inst_param_in"=w787) -> ("Readout parameters out"=w784:T12)
                          n326 = local write "Readout parameters"(w784) -> ()
                        }
                        frame 12 {
                          n327 = call "DSPClearBuffer.vi"("Inst info"=w788, "ramp?"=w789) -> ()  [unwired: 1 in]
                        }
                        frame 100, Default {
                        }
                      }
                    }
                    n328 = local read "Timings"() -> (w774:dbl[][])
                    n329 = Enqueue Element(queue=w776, element=w777) -> ()  [unwired: 2 in, 3 out]
                    n330 = Tick Count (ms)() -> (millisecond timer value=w770:u32)
                    n331 = call "Timer.vi"("index"=13, "Timings in"=w774, "t1"=w772, "t2"=w770) -> ("Timings out"=w773:dbl[][])  [unwired: 2 in]
                    n332 = local write "Timings"(w773) -> ()
                  }
                  frame #7 {
                    # "Add data to plot queue"
                    n333 = local read "Plot parameters"() -> (w800:T2)
                    n334 = local read "Timings"() -> (w793:dbl[][])
                    n335 = Tick Count (ms)() -> (millisecond timer value=w790:u32)
                    n336 = call "Timer.vi"("index"=15, "Timings in"=w793, "t1"=w791, "t2"=w790) -> ("Timings out"=w792:dbl[][])  [unwired: 2 in]
                    n337 = Unbundle By Name(w800) -> ("Disable plot"=w795:bool)
                    n338 = case shown="False" w795 {
                      tunnel: w799 -> [w805 _]
                      tunnel: w798 -> [w804 _]
                      tunnel: w797 -> [w801 _]
                      tunnel: w796 -> [w803 _]
                      frame False {
                        n339 = local read "Plot parameters"() -> (w807:T2)
                        n340 = call "Plot_add_to_buffer.vi"("Plot parameters in"=w807, "fast mode"=enum16{"normal sweep", "fast sweep"}."fast sweep", "Points"=w803, "new_data"=w801, "sweep_dim"=w804, "Indexes"=w805) -> ("Plot parameters out"=w806:T2)  [unwired: 1 in]
                        n341 = local write "Plot parameters"(w806) -> ()
                      }
                      frame True {
                      }
                    }
                    n342 = local write "Timings"(w792) -> ()
                  }
                  frame #8 {
                    # "meas loop time"
                    n343 = local read "Timings"() -> (w820:dbl[][])
                    n344 = Tick Count (ms)() -> (millisecond timer value=w812:u32)
                    n345 = call "Timer.vi"("index"=2, "Timings in"=w820, "t1"=w809, "t2"=w812) -> ("Timings out"=w811:dbl[][])  [unwired: 2 in]
                    n346 = Tick Count (ms)() -> (millisecond timer value=w813:u32)
                    n347 = call "Timer.vi"("index"=9, "Timings in"=w811, "t1"=w808, "t2"=w813) -> ("Timings out"=w814:dbl[][])  [unwired: 2 in]
                    n348 = local write "Timings"(w814) -> ()
                    n349 = call "RemainingTime.vi"("Timings"=w814, "sweep_dim"=w816, "Count"=w815) -> ("Remaning time (min)"=→"Remaning time (min)":dbl)
                  }
                }
                n350 = local write "Indexes"(w699) -> ()
                n351 = Increment(x=w695) -> (x+1=w708:u64)
                n352 = local read "Stop"() -> (w682:bool)
                n353 = Decrement(x=w683) -> (x-1=w706:u64[])
                n354 = Equal?(x=w704, y=w706) -> (x = y?=w707:bool)
                n355 = Or(x=w707, y=w682) -> (x .or. y?=w686:bool)
              }
              n356 = local read "Timings"() -> (w667:dbl[][])
              n357 = Tick Count (ms)() -> (millisecond timer value=w664:u32)
              n358 = call "Timer.vi"("index"=8, "Timings in"=w667, "t1"=w663, "t2"=w664) -> ("Timings out"=w666:dbl[][])  [unwired: 2 in]
              n359 = local write "Timings"(w666) -> ()
            }
            frame #6 {
              # "Post sweep treatment for the readout instruments"
              # "Final wait and close ADC etc."
              n360 = local read "Readout parameters"() -> (w821:T12)
              n361 = call "DAC_wait_end-of-move.vi"("FPGA VI Reference In"=w822) -> ()  [unwired: 1 in, 10 out]
              n362 = for {
                tunnel: w821 -> [w823] mode=indexing
                n363 = Unbundle By Name(w823) -> ("Kind"=w824:u16)
                n364 = case shown="0" w824 {
                  tunnel: w823 -> [w830 _]
                  frame 0 {
                    w829 = 0
                    n365 = Unbundle By Name(w830) -> ("DAQmx take out list"=w827:refnum<k21>[])
                    n366 = Increment(x=w829) -> (x+1=w828:i32)
                    n367 = Index Array(array=w827, index=w829) -> (element=w826:refnum<k21>)
                    n368 = Index Array(array=w827, index=w828) -> (element=w825:refnum<k21>)
                    n369 = call <vilib>:"DAQmx Clear Task.vi"("task in"=w826) -> ()  [unwired: 14 in, 1 out]
                    n370 = call <vilib>:"DAQmx Clear Task.vi"("task in"=w825) -> ()  [unwired: 14 in, 1 out]
                  }
                  frame 100, Default {
                  }
                }
              }
            }
          }
        }
      }
    }
    frame #3 {
      # "Post measurement treatment (temporal because it is not so nice.)"
      # "Go back to the initial position if it is required."
      n371 = local read "Exp_params"() -> (w839:T15)
      n372 = Unbundle By Name(w839) -> ("Experimental bool list"=w840:bool[], "FPGA Ref"=w841:T14)
      n373 = Index Array(array=w840, index=0) -> (element=w842:bool)
      n374 = Unbundle By Name(w839) -> ("Inst_parameters.Inst_array"=w834:T12, "Read out instrument bools"=w835:u64[][], "Sweep instrument bools"=w838:u64[][])
      n375 = case shown="True" w842 {
        tunnel: w839 -> [_ w851]
        tunnel: w841 -> [_ w850]
        tunnel: w840 -> [_ w848]
        tunnel: w831 -> [_ w844]
        frame False {
        }
        frame True {
          # "Move"
          # "Get initial values of sweep"
          # "Go to initial position"
          n376 = Unbundle By Name(w851) -> ("sweep_dim"=w854:u64[], "sweep_list"=w853:string[])
          n377 = call "Count2Indexes.vi"("sweep_dim"=w854, "Count"=0) -> ("Indexes"=w845:u64[])
          n378 = local read "Sweep inst info"() -> (w846:T12)
          n379 = call "GetValueFromIndexes.vi"("sweep_list"=w853, "WorkFilePath"=w844, "Sweep inst info"=w846, "Indexes"=w845) -> ("Points"=w852:cluster{"name":string, "data":u64, "data":dbl}[])
          n380 = Index Array(array=w848, index=1) -> (element=w847:bool)
          n381 = call "Move.vi"("Points"=w852, "Sweep inst info"=w846, "FPGA Ref"=w850, "Use FPGA?"=w847, "WorkFilePath"=w844, "Indexes"=w845) -> ()  [unwired: 4 in, 1 out]
        }
      }
      n382 = Index Array(array=w838, index (col)=1) -> (element=w832:u64[])  [unwired: 1 in]
      n383 = Index Array(array=w835, index (col)=1) -> (element=w833:u64[])  [unwired: 1 in]
      n384 = call "Insts_post.vi"("Initialize sweep instruments ??"=w832, "Initialize readout instruments??"=w833, "Inst_array"=w834) -> ()  [unwired: 3 in]
    }
    frame #4 {
      n385 = local read "Indexes"() -> (w856:i32[])
      n386 = local read "Exp_params"() -> (w861:T15)
      n387 = Unbundle By Name(w861) -> ("Experimental bool list"=w859:bool[], "FPGA Ref"=w860:T14)
      n388 = Index Array(array=w859, index=1) -> (element=w858:bool)
      n389 = case shown="True" w858 {
        tunnel: w860 -> [_ w862]
        frame False {
        }
        frame True {
          # "Close FPGA"
          n390 = xnode "Close FPGA VI Reference"("FPGA VI Reference In"=w862) -> ()  [unwired: 1 in, 1 out]
        }
      }
    }
  }
  n391 = stacked-sequence {
    tunnel: w9 -> [w866 _ _]
    tunnel: w8 -> [w873 w894 _]
    tunnel: w2 -> [w875 _ _]
    tunnel: w1 -> [w874 _ _]
    frame #0 {
      # "Write final indexes of the sweep."
      n392 = call "GetTempFilePath.vi"("ExpFilePath"=w873) -> ("Temp file path"=w872:path)
      n393 = call <vilib>:"H5Fopen.vi"("mode (read-only)"=H5Fmode."open or create" ("mode"), "path"=w872) -> ("error out"=w865:errorcluster, "ref out"=w867:T13)  [unwired: 8 in]
      n394 = xnode "H5Awrite.xnode"("replace? (T)"=TRUE, "object name"="Param_list", "error in (no error)"=w865, "data"=w866, "attrib name"="sweep_index", "ref in"=w867) -> ("error out"=w864:errorcluster, "ref out"=w863:T13)  [unwired: 1 in, 1 out]
      n395 = call <vilib>:"H5Fclose.vi"("error in (no error)"=w864, "ref"=w863) -> ()  [unwired: 9 in, 1 out]
      n396 = Release Queue(queue=w874) -> ()  [unwired: 2 in, 3 out]
      n397 = Release Queue(queue=w875) -> ()  [unwired: 2 in, 3 out]
    }
    frame #1 {
      # "Finally copy temp file\nto actual file"
      n398 = Delete(path (use dialog)=w894) -> (error out=w896:errorcluster)  [unwired: 4 in, 2 out]
      n399 = call "GetTempFilePath.vi"("ExpFilePath"=w894) -> ("Temp file path"=w895:path)
      n400 = Unbundle By Name(w896) -> ("status"=w897:bool)
      n401 = case shown="True" w897 {
        tunnel: w895 -> [w898 _]
        tunnel: w894 -> [w900 _]
        frame False {
          n402 = call "repack-h5.vi"("dest"=w900, "source"=w898) -> ("error out"=w899:errorcluster)  [unwired: 1 in]
          n403 = Delete(path (use dialog)=w898, error in=w899) -> ()  [unwired: 3 in, 3 out]
        }
        frame True {
        }
      }
    }
    frame #2 {
      n404 = local write "Finish"(TRUE) -> ()
    }
  }
  n405 = while {
    stop <- w902 stop-if-true
    n406 = stacked-sequence {
      seq-local: [w903 _ _] -> [_ _ w947]
      frame #0 {
        n407 = Tick Count (ms)() -> (millisecond timer value=w903:u32)
      }
      frame #1 {
        n408 = local read "Plot parameters"() -> (w904:T2)
        n409 = Unbundle By Name(w904) -> ("Disable plot"=w905:bool)
        n410 = case shown="False" w905 {
          tunnel: w904 -> [w916 _]
          frame False {
            # "Plot loop"
            n411 = Unbundle By Name(w916) -> ("Sweep buffer"=w919:dbl[][], "Readout buffer"=w918:dbl[][], "Xparameter"=w908:dbl, "Channel"=w914:dbl)
            n412 = local read "Exp_params"() -> (w915:T15)
            n413 = Equal?(x=w908, y=0.0) -> (x = y?=w913:bool)
            n414 = Decrement(x=w908) -> (x-1=w909:dbl)
            n415 = case shown="True" w913 {
              tunnel: w915 -> [w932 w941]
              tunnel: w914 -> [w931 w940]
              tunnel: w909 -> [w922 w935]
              tunnel: [w921 "counter"] -> w910
              tunnel: [w920 w934] -> w911
              frame False {
                n416 = call "Plot_build_legend.vi"("Y_id"=w931, "X_id"=w922, "Exp_params"=w932) -> ("Yunit"=w923:string, "Yname"=w924:string, "Xunit"=w925:string, "Xname"=w928:string)  [unwired: 3 in]
                n417 = Concatenate Strings(w924, " (", w923, ")") -> (w920:string)
                n418 = Concatenate Strings(w928, " (", w925, ")") -> (w921:string)
              }
              frame True {
                n419 = call "Plot_build_legend.vi"("Y_id"=w940, "X_id"=w935, "Exp_params"=w941) -> ("Yunit"=w936:string, "Yname"=w937:string)  [unwired: 3 in, 2 out]
                n420 = Concatenate Strings(w937, " (", w936, ")") -> (w934:string)
              }
            }
            n421 = Index Array(array=w918, index (col)=w914) -> (element=w906:dbl[])  [unwired: 1 in]
            n422 = Index Array(array=w919, index (col)=w908) -> (element=w907:dbl[])  [unwired: 1 in]
            n423 = Bundle("Sweep buffer"=w907, "Readout buffer"=w906) -> (→"Graph":T1)  [unwired: 1 in]
            n424 = property on="Graph" class="XYGraph (strict)"("YScale.NameLbl.Text"=w911) -> ()  [unwired: 2 in, 2 out]
            n425 = property on="Graph" class="XYGraph (strict)"("XScale.NameLbl.Text"=w910) -> ()  [unwired: 2 in, 2 out]
          }
          frame True {
          }
        }
      }
      frame #2 {
        n426 = local read "Timings"() -> (w946:dbl[][])
        n427 = Tick Count (ms)() -> (millisecond timer value=w943:u32)
        n428 = call "Timer.vi"("index"=2, "Timings in"=w946, "t1"=w947, "t2"=w943) -> ("Timings out"=w945:dbl[][])  [unwired: 2 in]
        n429 = local write "Timings"(w945) -> ()
        n430 = Wait (ms)(milliseconds to wait=100) -> ()  [unwired: 1 out]
      }
    }
    n431 = local read "Finish"() -> (w902:bool)
  }
